vi "Auto_New.vi"() -> ()   [LabVIEW 2017]
uses:
  Control/Saurabh/prosucer_consumer_enum1.ctl
  Control/OUTPUT Cluster Indicator.ctl
  <vilib>/Utility/error.llb/DialogType.ctl
  <vilib>/addons/database/Connection.llb/DB Tools Open Connec (String).vi
  Global/DATA LOG.vi
  Global/Global 1.vi
  <vilib>/addons/database/NI_Database_API.lvlib
panel:
  out "SHIFT":string
  in  "BARCODE RECIPE":string(combo)
  out "PLC COM.":bool
  out "SHIFT_DATA":string[](array[string])
  out "stop":bool
  out "error out 2":errorcluster
  out "Shift 4":i32
  out "Time Stamp Out":timestamp[](array[timestamp]) format="%<%X>T"
  out "Time Stamp Out 4":timestamp[](array[timestamp]) format="%<%X>T"
  out "Shift_change":bool
  out "appended array":string[][](array[string])
  out "SHIFT_DATA 2":string[](array[string])
  in  "error in (no error)":errorcluster
  in  "Tab Control":enum32{"Screen 1", "Screen 2", "Daignostic"}(tab)
  out "OP 50":bool
  out "OP 40":bool
  out "OP 30":bool
  out "OP - 50":T1 {"RH Motor Screw" format="%#.2g N-m"; "LH Motor Screw" format="%#.2g N-m"; "Nut Torque" format="%#.2g N-m"}
  out "OP - 40":T2 {"Stack Load" format="%.2f kg"; "Dispalcement" format="%#.2g mm"; "LH Screw" format="%#.2g N-m"; "RH Screw" format="%#.2g N-m"}
  out "OP - 30":T3 {"Shaft Press Load" format="%#.2g kg"; "Displacement" format="%#.2g mm"}
  in  "stop 2":bool
  out "OP - 10":T4 {"Leak Rate" format="%#.2g SCCM"}
  in  "SIMULATE INPUT":bool[](array[boolean])=[FALSE, FALSE, FALSE, FALSE]
  out "OP - 20":T5 {"Top Load" format="%#.2g kg"; "Top Displace" format="%#.2g mm"; "Bottom Load" format="%#.2g kg"; "Bottom Displace" format="%#.2g mm"}
  out "OP 10 & 20":bool
  out "OP - 60":T6 {"Screw 6" format="%#.2g N-m"; "Screw 5" format="%#.2g N-m"; "Screw 4" format="%#.2g N-m"; "Screw 3" format="%#.2g N-m"; "Screw 2" format="%#.2g N-m"; "Screw 1" format="%#.2g N-m"}
  out "OP - 70":T7 {"Full Open" format="%#.4g V"; "Full Close" format="%#.4g V"}
  out "OP - 110":cluster{"BARCODE":string}
  out "OP - 80":T8 {"Plug Press Load" format="%#.2f kg"}
  out "OP - 90":T9 {"Steam Leak" format="%#_g sccm"; "Seat Leak" format="%#_g LPM"}
  out "OP - 100":T10 {"Response Time REV" format="%#_g msec"; "Response time FWD" format="%#_g msec"; "Motor Full Open" format="%#.2f V"; "Motor Start Back" format="%#.2f V"; "Motor Full Close" format="%#.2f V"; "Motor Start Of Close" format="%#.2f V"; "Motor Peak" format="%#.2f A"; "Sensor O/P Full Close" format="%#.2f V"; "Sensor O/P Start Of Close" format="%#.2f V"; "Sensor O/P Open" format="%#.2f V"}
  out "OP 60":bool
  out "OP 70 & 80":bool
  out "OP 90 -100 - 110":bool
  out "OP110 STATUS":dbl[](array[numeric])
  out "SCAN OP110":string[](array[string])
  out "OP100 STATUS":dbl[](array[numeric])
  out "SCAN OP100":string[](array[string])
  out "OP50 STATUS":dbl[](array[numeric])
  out "SCAN OP50":string[](array[string])
  out "OP90 STATUS":dbl[](array[numeric])
  out "SCAN OP90":string[](array[string])
  out "OP80 STATUS":dbl[](array[numeric])
  out "SCAN OP80":string[](array[string])
  out "OP70 STATUS":dbl[](array[numeric])
  out "SCAN OP70":string[](array[string])
  out "OP60 STATUS":dbl[](array[numeric])
  out "SCAN OP60":string[](array[string])
  out "OP40 STATUS":dbl[](array[numeric])
  out "SCAN OP40":string[](array[string])
  out "OP30 STATUS":dbl[](array[numeric])
  out "SCAN OP30":string[](array[string])
  out "OP20 STATUS":dbl[](array[numeric])
  out "SCAN OP20":string[](array[string])
  out "OP10 STATUS":dbl[](array[numeric])
  out "SCAN OP10":string[](array[string])
  # "Op10 20\nOp30\nOp 40\nOp50\nOp60\nOp70-80\nOp 90-100-110"
  # "SENSOR MIN VLTG"
  # "OP - 50"
  # "OP - 40"
  # "OP - 30"
  # "OP - 10"
  # "OP - 20"
  # "OP - 60"
  # "OP - 70"
  # "OP - 110"
  # "OP - 80"
  # "OP - 90"
  # "OP - 100"
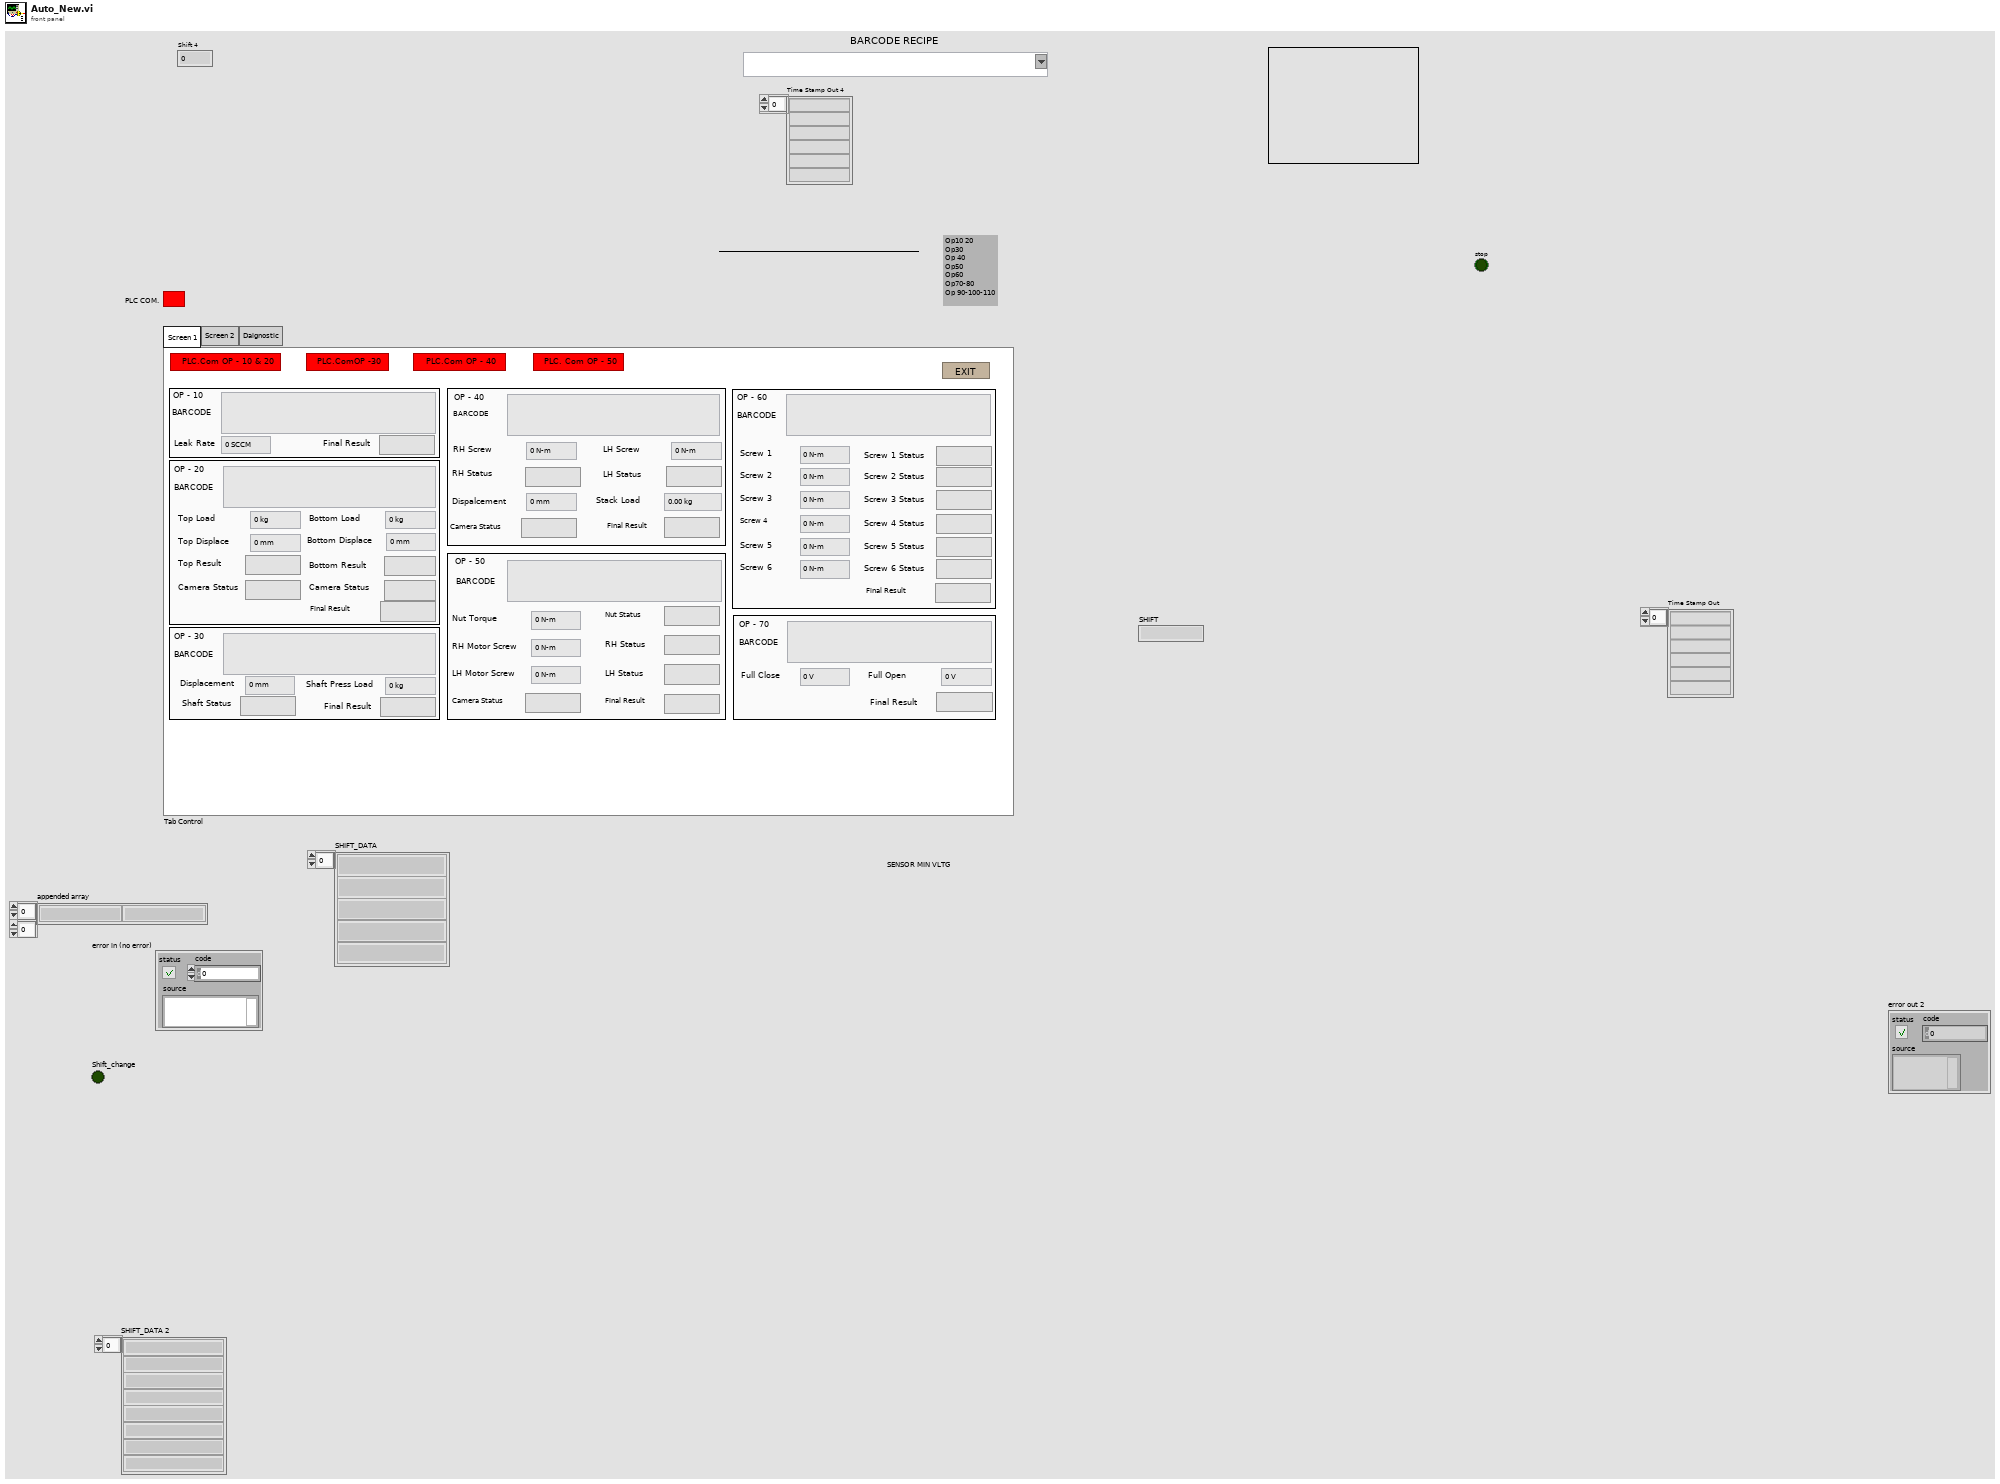
[diagram p1: front panel]
types:
  T1 = cluster{"BARCODE":string, "Nut Torque":dbl, "LH Motor Screw":dbl, "LH Status":bool, "RH Status":bool, "RH Motor Screw":dbl, "Final Result":bool, "Nut Status":bool, "Camera Status":bool}
  T2 = cluster{"BARCODE":string, "RH Screw":dbl, "LH Screw ":dbl, "RH Status":bool, "LH Status":bool, "Dispalcement ":dbl, "Stack Load ":dbl, "Final Result":bool, "Camera Status":bool}
  T3 = cluster{"BARCODE":string, "Displacement":dbl, "Shaft Press Load":dbl, "Shaft Status":bool, "Final Result":bool}
  T4 = cluster{"BARCODE":string, "Leak Rate":dbl, "Final Result":bool}
  T5 = cluster{"BARCODE":string, "Bottom Displace":dbl, "Bottom Load":dbl, "Camera Status":bool, "Bottom Result":bool, "Top Displace":dbl, "Top Load ":dbl, "Camera Status":bool, "Top Result":bool, "Final Result":bool}
  T6 = cluster{"BARCODE":string, "Screw 1":dbl, "Screw 2":dbl, "Screw 1 Status":bool, "Screw 2 Status":bool, "Screw 3":dbl, "Final Result":bool, "Screw 3 Status":bool, "Screw 4":dbl, "Screw 5":dbl, "Screw 4 Status":bool, "Screw 5 Status":bool, "Screw 6":dbl, "Screw 6 Status":bool}
  T7 = cluster{"BARCODE":string, "Full Close":dbl, "Full Open":dbl, "Final Result":bool}
  T8 = cluster{"BARCODE":string, "Plug Press Load":dbl, "Final Result":bool, "Loctite Status":bool}
  T9 = cluster{"BARCODE":string, "Seat Leak":dbl, "Seat Status":bool, "Steam Leak":dbl, "Final Result":bool}
  T10 = cluster{"BARCODE":string, "Sensor O/P Open":dbl, "Sensor O/P Start Of Close":dbl, "Final Result":bool, "Sensor O/P Full Close":dbl, "Motor Peak":dbl, "Motor Start Of Close":dbl, "Motor Full Close":dbl, "Motor Start Back":dbl, "Motor Full Open":dbl, "Response time FWD":dbl, "Response Time REV":dbl, "Camera Status":bool}
  T11 = typedef "OUTPUT Cluster Indicator.ctl" = cluster{"OP - 10":cluster{"BARCODE":string, "LEAK RATE":dbl, "RESULT":bool}, "OP - 30":cluster{"BARCODE":string, "Displacement":dbl, "Load":dbl, "Middle Gear Shaft Status":bool, "Final Result":bool}, "OP - 60":cluster{"BARCODE":string, "Screw 1 Data":dbl, "Screw 2 data":dbl, "Screw 1 Status":bool, "Screw 2 Status":bool, "Screw3 Data":dbl, "Final Result":bool, "Screw3 Status":bool, "Screw4 Data":dbl, "Screw5 Data":dbl, "Screw4 Status":bool, "Screw5 Status":bool, "Screw6 Data":dbl, "Screw6 Status":bool}, "OP - 70":cluster{"BARCODE":string, "Sensor MIN Vltg":dbl, "Sensor MAX Vltg":dbl, "Final Result":bool}, "OP - 80":cluster{"BARCODE":string, "Load":dbl, "Final Result":bool, "Dispensing":bool}, "OP - 90":cluster{"BARCODE":string, "Seat LT Data":dbl, "Seat Status":bool, "Steam LT Data":dbl, "Final Result":bool}, "OP - 110":cluster{"BARCODE":string}, "OP - 20":cluster{"BARCODE":string, "Bottom Displace":dbl, "Bottom Load":dbl, "Camera Status":bool, "Bottom Result":bool, "Top Displace":dbl, "Top Load ":dbl, "Camera Status":bool, "Top Result":bool, "Final Result":bool}, "OP - 50":cluster{"BARCODE":string, "Nut Torque":dbl, "LH Motor Screw":dbl, "LH Status":bool, "RH Status":bool, "RH Motor Screw":dbl, "Final Result":bool, "Nut Status":bool, "Camera Status":bool}, "OP - 100":cluster{"BARCODE":string, "Sensor O/P Open":dbl, "Sensor O/P Start Of Close":dbl, "Final Result":bool, "Sensor O/P Full Close":dbl, "Motor Peak":dbl, "Motor Start Of Close":dbl, "Motor Full Close":dbl, "Motor Start Back":dbl, "Motor Full Open":dbl, "Response time FWD":dbl, "Response Time REV":dbl, "Camera Status":bool}, "OP - 40":cluster{"BARCODE":string, "RH Screw":dbl, "LH Screw ":dbl, "RH Status":bool, "LH Status":bool, "Dispalcement ":dbl, "Stack Load ":dbl, "Final Result":bool, "Camera Status":bool}}
  T12 = cluster{"OP - 10":cluster{"BARCODE":string, "LEAK RATE":dbl, "RESULT":bool}, "OP - 30":cluster{"BARCODE":string, "Displacement":dbl, "Load":dbl, "Middle Gear Shaft Status":bool, "Final Result":bool}, "OP - 60":cluster{"BARCODE":string, "Screw 1 Data":dbl, "Screw 2 data":dbl, "Screw 1 Status":bool, "Screw 2 Status":bool, "Screw3 Data":dbl, "Final Result":bool, "Screw3 Status":bool, "Screw4 Data":dbl, "Screw5 Data":dbl, "Screw4 Status":bool, "Screw5 Status":bool, "Screw6 Data":dbl, "Screw6 Status":bool}, "OP - 70":cluster{"BARCODE":string, "Sensor MIN Vltg":dbl, "Sensor MAX Vltg":dbl, "Final Result":bool}, "OP - 80":cluster{"BARCODE":string, "Load":dbl, "Final Result":bool, "Dispensing":bool}, "OP - 90":cluster{"BARCODE":string, "Seat LT Data":dbl, "Seat Status":bool, "Steam LT Data":dbl, "Final Result":bool}, "OP - 110":cluster{"BARCODE":string}, "OP - 20":cluster{"BARCODE":string, "Bottom Displace":dbl, "Bottom Load":dbl, "Camera Status":bool, "Bottom Result":bool, "Top Displace":dbl, "Top Load ":dbl, "Camera Status":bool, "Top Result":bool, "Final Result":bool}, "OP - 40":cluster{"BARCODE":string, "RH Screw":dbl, "LH Screw ":dbl, "RH Status":bool, "LH Status":bool, "Dispalcement ":dbl, "Stack Load ":dbl, "Final Result":bool}, "OP - 50":cluster{"BARCODE":string, "Nut Torque":dbl, "LH Motor Screw":dbl, "LH Status":bool, "RH Status":bool, "RH Motor Screw":dbl, "Final Result":bool, "Nut Status":bool, "Camera Status":bool}, "OP - 100":cluster{"BARCODE":string, "Sensor O/P Open":dbl, "Sensor O/P Start Of Close":dbl, "Final Result":bool, "Sensor O/P Full Close":dbl, "Motor Peak":dbl, "Motor Start Of Close":dbl, "Motor Full Close":dbl, "Motor Start Back":dbl, "Motor Full Open":dbl, "Response time FWD":dbl, "Response Time REV":dbl, "Camera Status":bool}}
  T13 = typedef "prosucer_consumer_enum1.ctl" = enum16{"-1", "SCAN1", "SCAN2", "SCAN3", "SCAN4", "SCAN5", "SCAN6", "SCAN7", "SCAN8", "SCAN9", "SCAN10", "SCAN11", "STOP", "DATALOG1", "DATALOG2", "DATALOG3", "DATALOG4", "DATALOG5", "DATALOG6", "DATALOG7", "DATALOG8", "DATALOG9", "DATALOG10", "DATALOG11", "CYCLE_START1", "CYCLE_START2", "CYCLE_START3", "CYCLE_START4", "BARCODE RECIPE", "EMERGENCY STOP"}
  T14 = typedef "NI_Database_API.lvlib/Conn ObjectReference.ctl" = refnum<k1>
  T15 = typedef "DialogType.ctl" = u16
  T16 = cluster{"trimmed string":string, "SHIFT":string, "date/time string":string, string, "Input 2":string}
  T17 = cluster{"SHIFT":string, "date/time string":string, "Input 2":string, string}
  T18 = cluster{"date/time string":string, "Input 2":string, "Input 2":string, "Input 2":string, "Input 2":string, "Input 2":string, "Input 2":string, "Input 2":string, "Input 2":string, "Input 2":string, "Input 2":string}
  T19 = cluster{"date/time string":string, "SHIFT":string, "Input 2":string, "Input 2":string, "Input 2":string, "Input 2":string, "Input 2":string, "Input 2":string, "Input 2":string, "Input 2":string, "Input 2":string, "Input 2":string}
  T20 = cluster{"date/time string":string, "Input 2":string, "Input 2":string, "Input 2":string, "Input 2":string}
  T21 = cluster{"date/time string":string, "SHIFT":string, "Input 2":string, "Input 2":string, "Input 2":string, "Input 2":string}
  T22 = cluster{"date/time string":string, "Input 2":string, "Input 2":string, "Input 2":string, "Input 2":string, "Input 2":string, "Input 2":string, "Input 2":string, "Input 2":string}
  T23 = cluster{"date/time string":string, "SHIFT":string, "Input 2":string, "Input 2":string, "Input 2":string, "Input 2":string, "Input 2":string, "Input 2":string, "Input 2":string, "Input 2":string}
  T24 = cluster{"date/time string":string, "SHIFT":string, "Input 2":string, "Input 2":string, "Input 2":string, "Input 2":string, "Input 2":string, "Input 2":string}
  T25 = cluster{"date/time string":string, "Input 2":string, "Input 2":string, "Input 2":string, "Input 2":string, "Input 2":string, "Input 2":string, "Input 2":string, "Input 2":string, "Input 2":string, "Input 2":string, "Input 2":string, "Input 2":string, "Input 2":string}
  T26 = cluster{"date/time string":string, "SHIFT":string, "Input 2":string, "Input 2":string, "Input 2":string, "Input 2":string, "Input 2":string, "Input 2":string, "Input 2":string, "Input 2":string, "Input 2":string, "Input 2":string, "Input 2":string, "Input 2":string}
  T27 = cluster{"date/time string":string, "Input 2":string, "Input 2":string, "Input 2":string}
  T28 = cluster{"date/time string":string, "SHIFT":string, "Input 2":string, "Input 2":string, "Input 2":string}
  T29 = cluster{"Input 2":string, "SHIFT":string, "date/time string":string, "Input 2":string, "Input 2":string, "Input 2":string}
  T30 = cluster{"BARCODE":string, "Seat LT Data":dbl, "Seat Status":bool, "Steam LT Data":dbl, "Final Result":bool}
  T31 = cluster{"BARCODE":string, "LEAK RATE":dbl, "RESULT":bool}
  T32 = cluster{"BARCODE":string, "Displacement":dbl, "Load":dbl, "Middle Gear Shaft Status":bool, "Final Result":bool}
  T33 = cluster{"BARCODE":string, "Screw 1 Data":dbl, "Screw 2 data":dbl, "Screw 1 Status":bool, "Screw 2 Status":bool, "Screw3 Data":dbl, "Final Result":bool, "Screw3 Status":bool, "Screw4 Data":dbl, "Screw5 Data":dbl, "Screw4 Status":bool, "Screw5 Status":bool, "Screw6 Data":dbl, "Screw6 Status":bool}
  T34 = cluster{"BARCODE":string, "Sensor MIN Vltg":dbl, "Sensor MAX Vltg":dbl, "Final Result":bool}
  T35 = cluster{"BARCODE":string, "Load":dbl, "Final Result":bool, "Dispensing":bool}
  T36 = enum32{"invalid app kind", "Development System", "Run Time System", "Student Edition", "Embedded LabVIEW", "Evaluation", "Custom"}
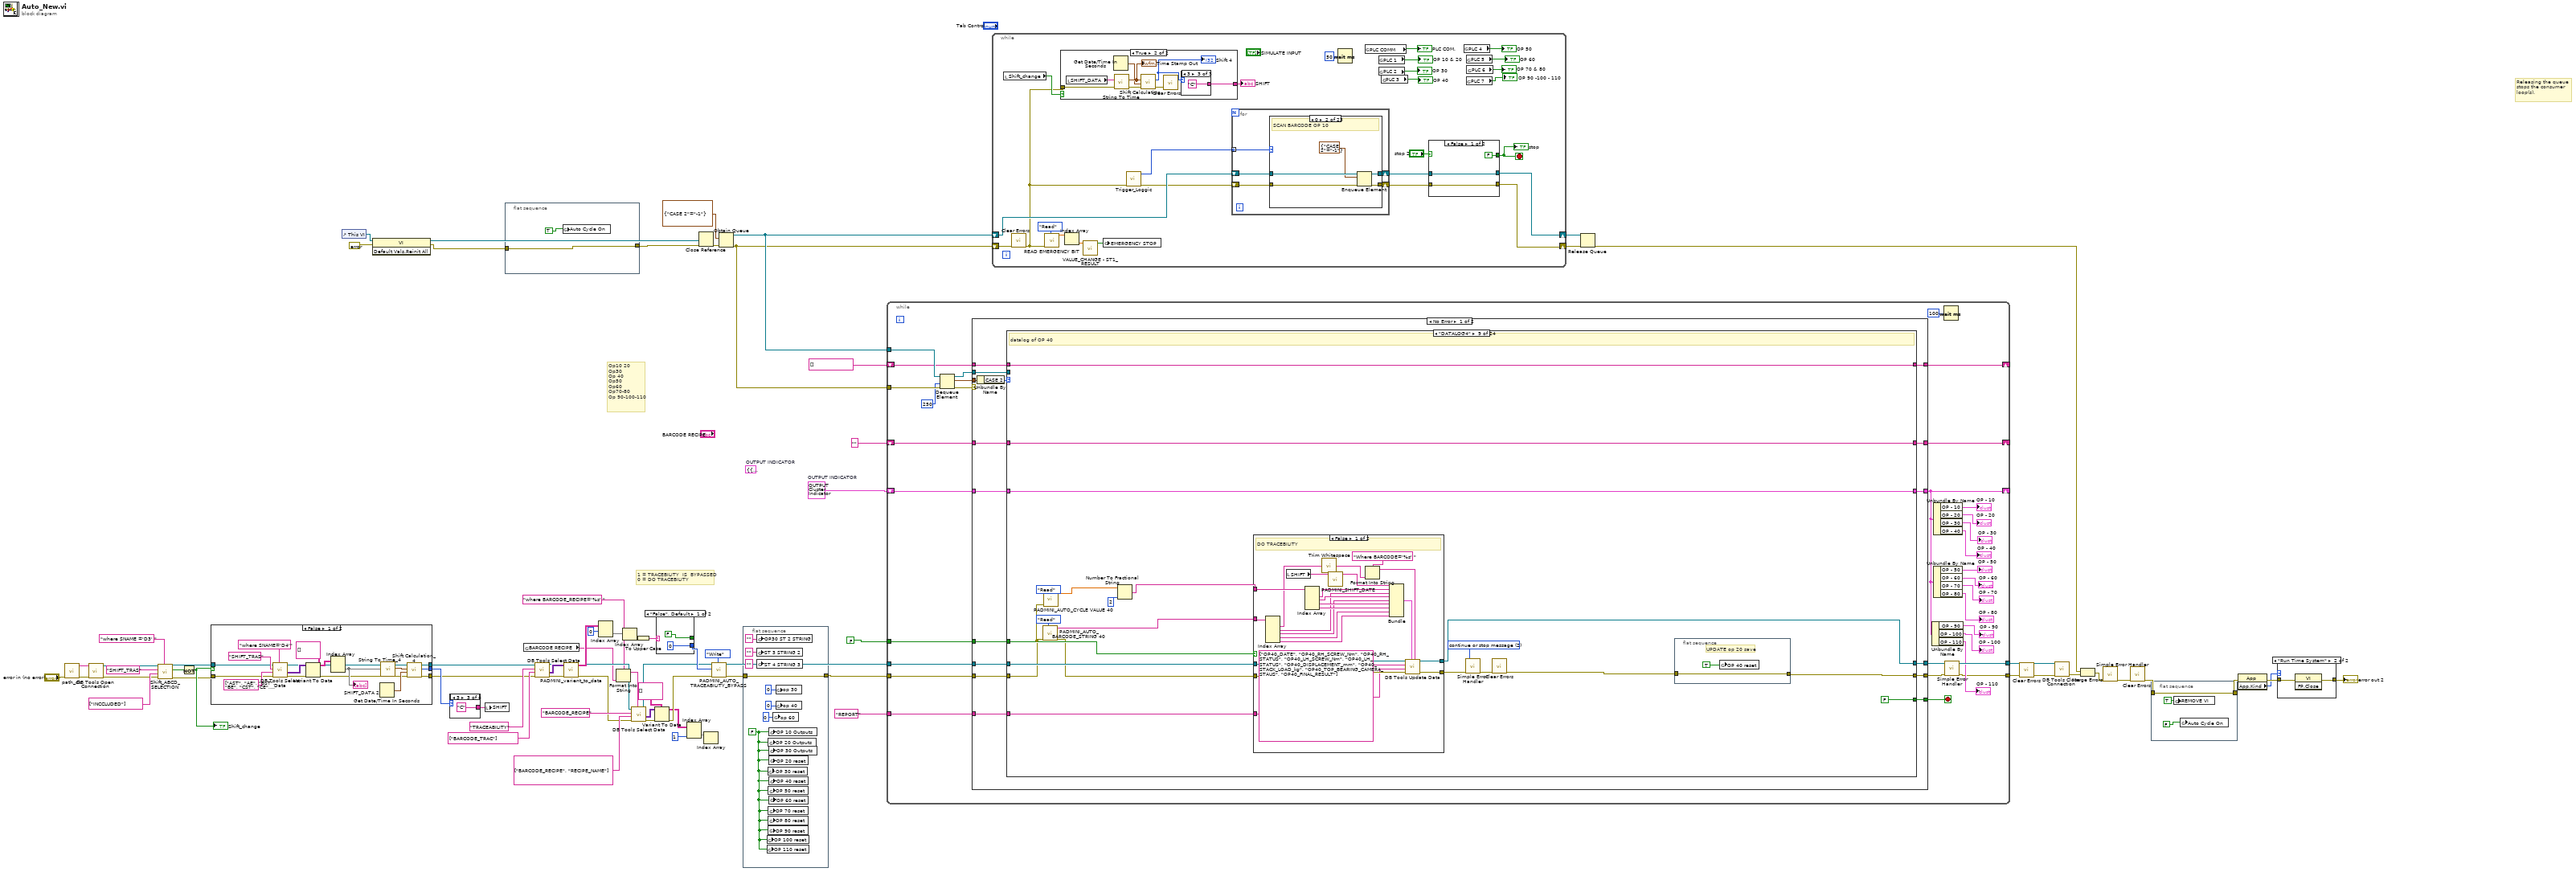
[diagram p0: block diagram]
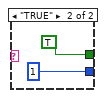
[diagram p2: hidden frame]
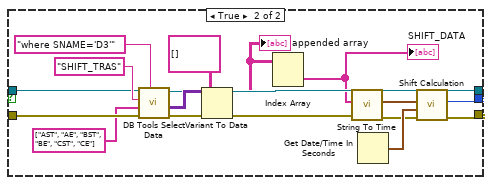
[diagram p3: hidden frame]
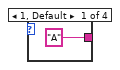
[diagram p4: hidden frame]
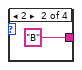
[diagram p5: hidden frame]
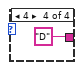
[diagram p6: hidden frame]
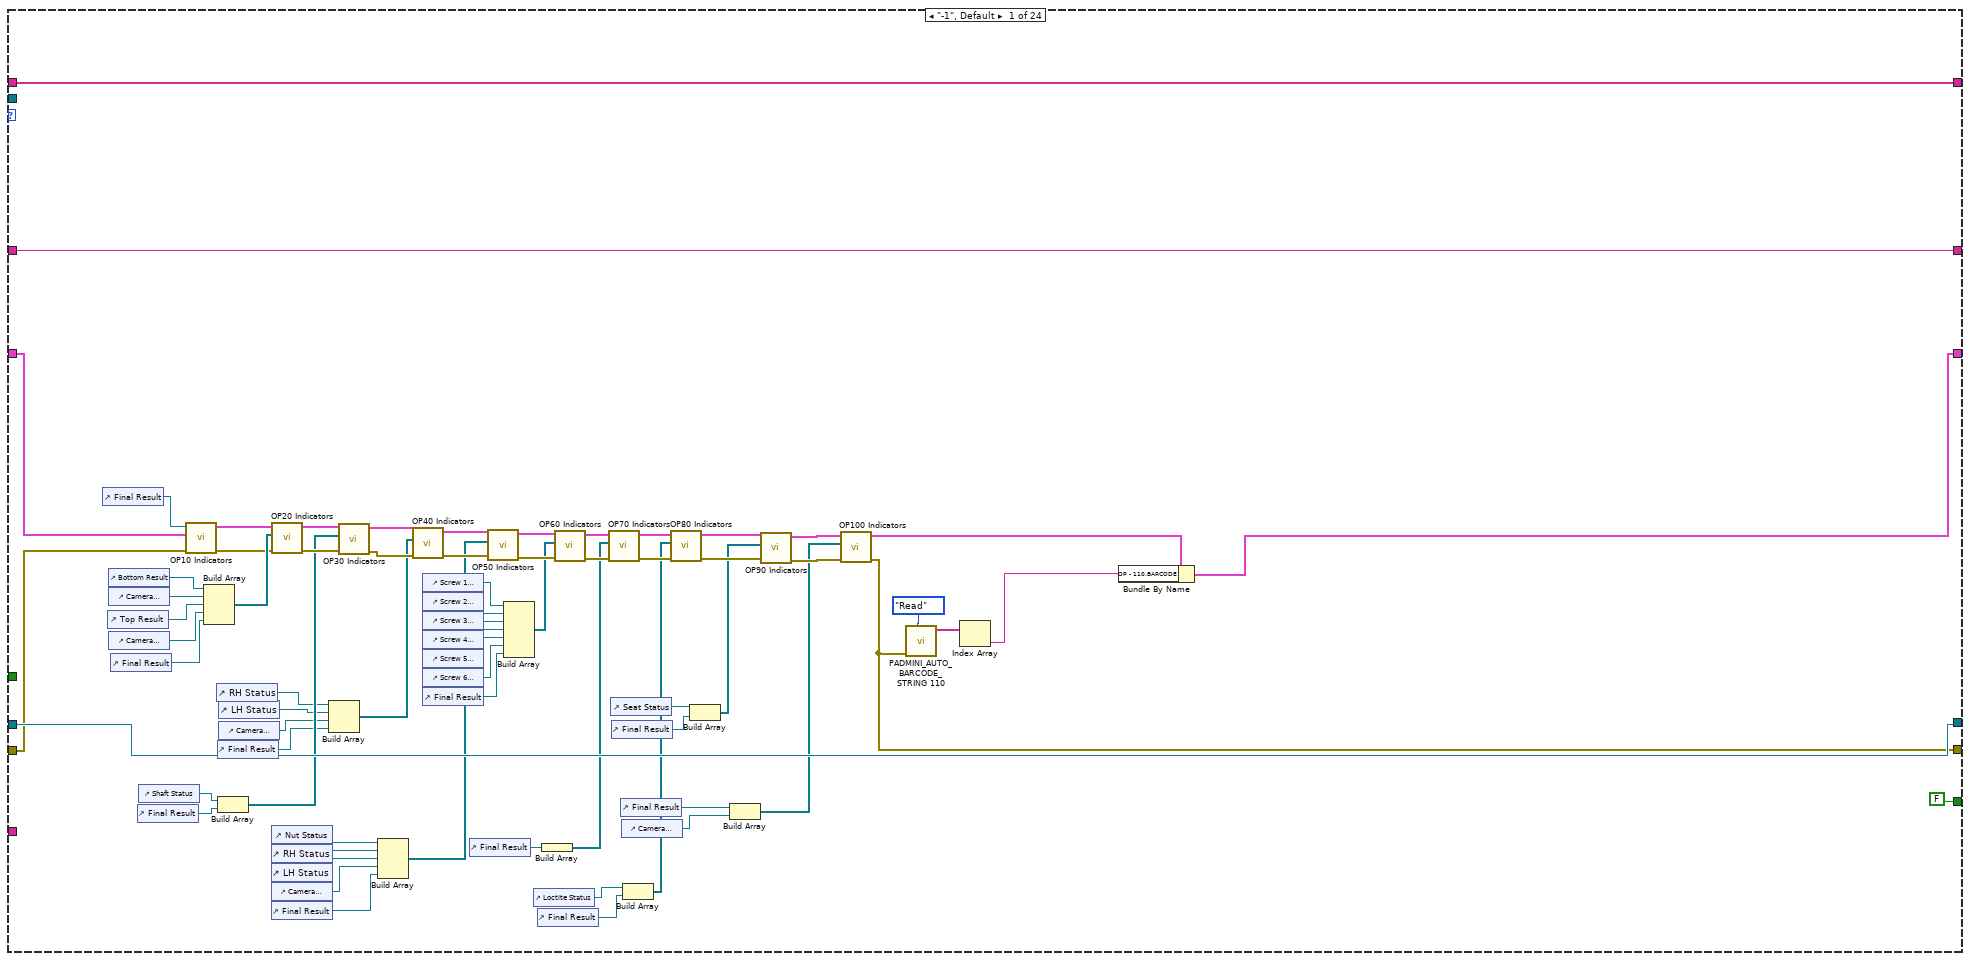
[diagram p7: hidden frame]
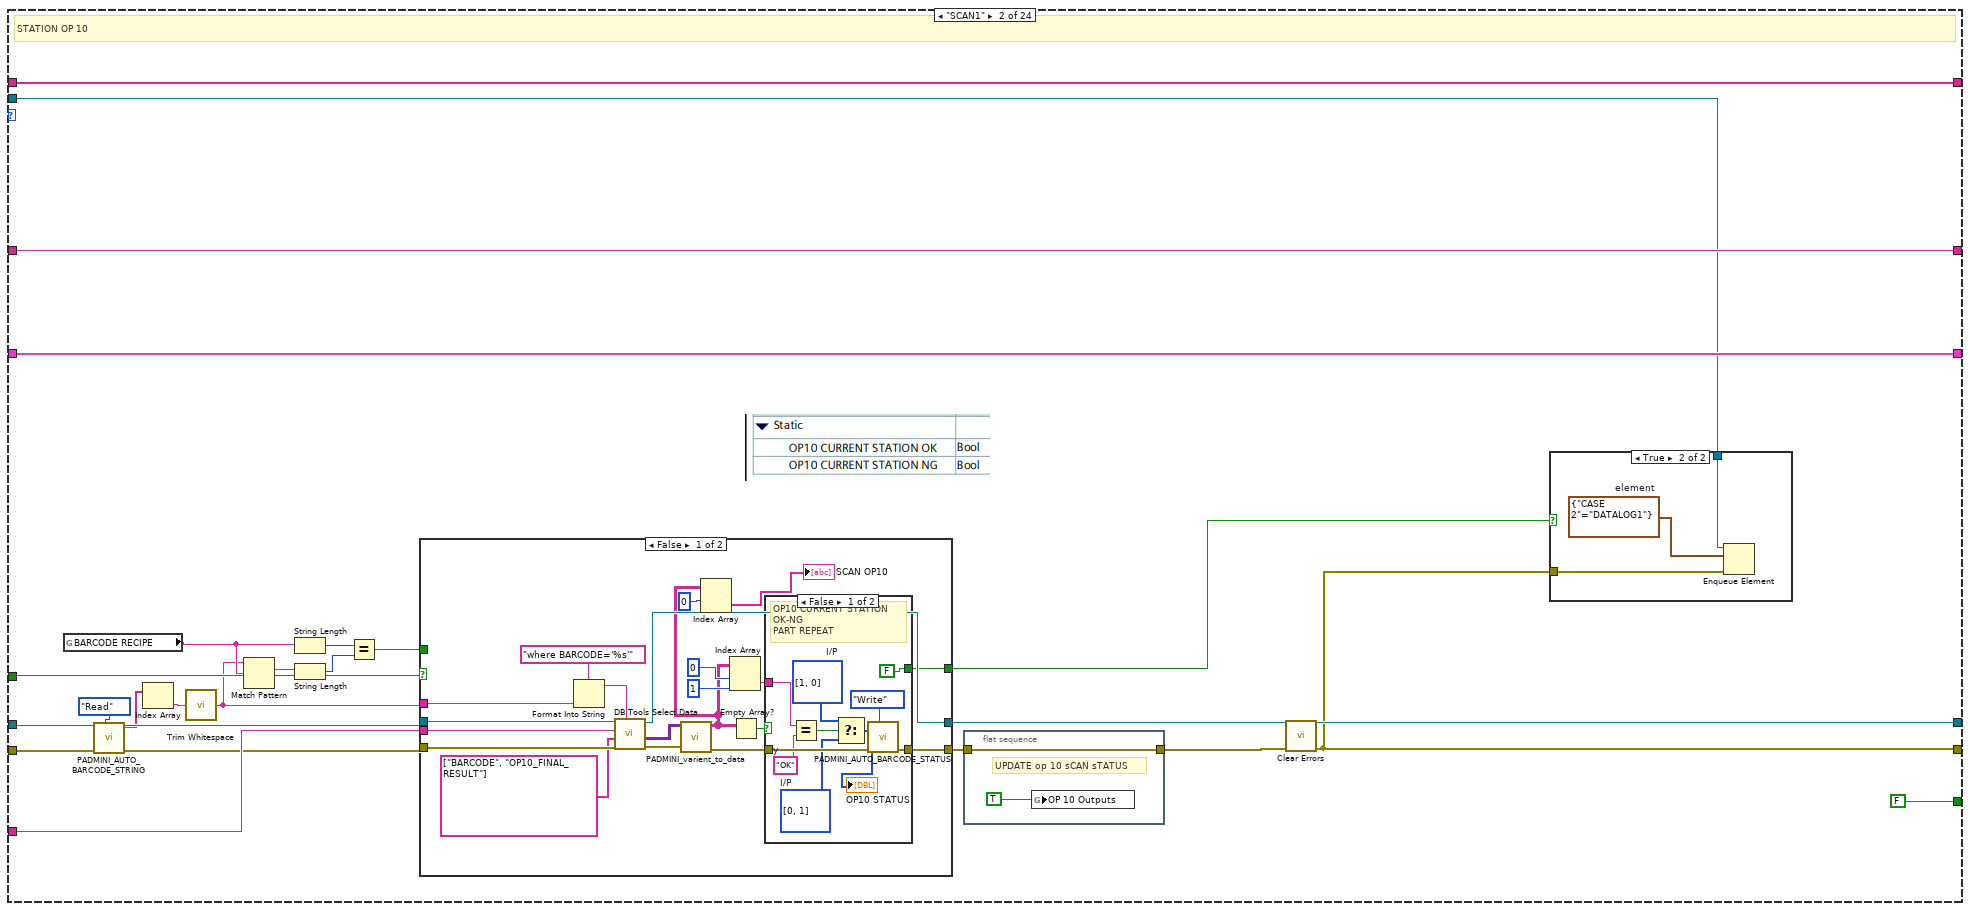
[diagram p8: hidden frame]
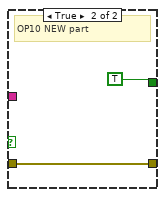
[diagram p10: hidden frame]
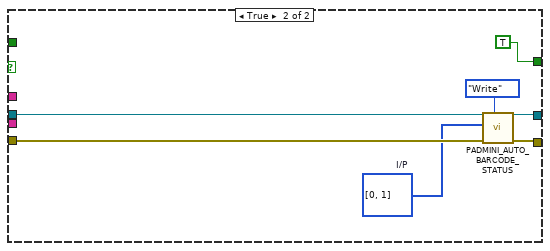
[diagram p11: hidden frame]
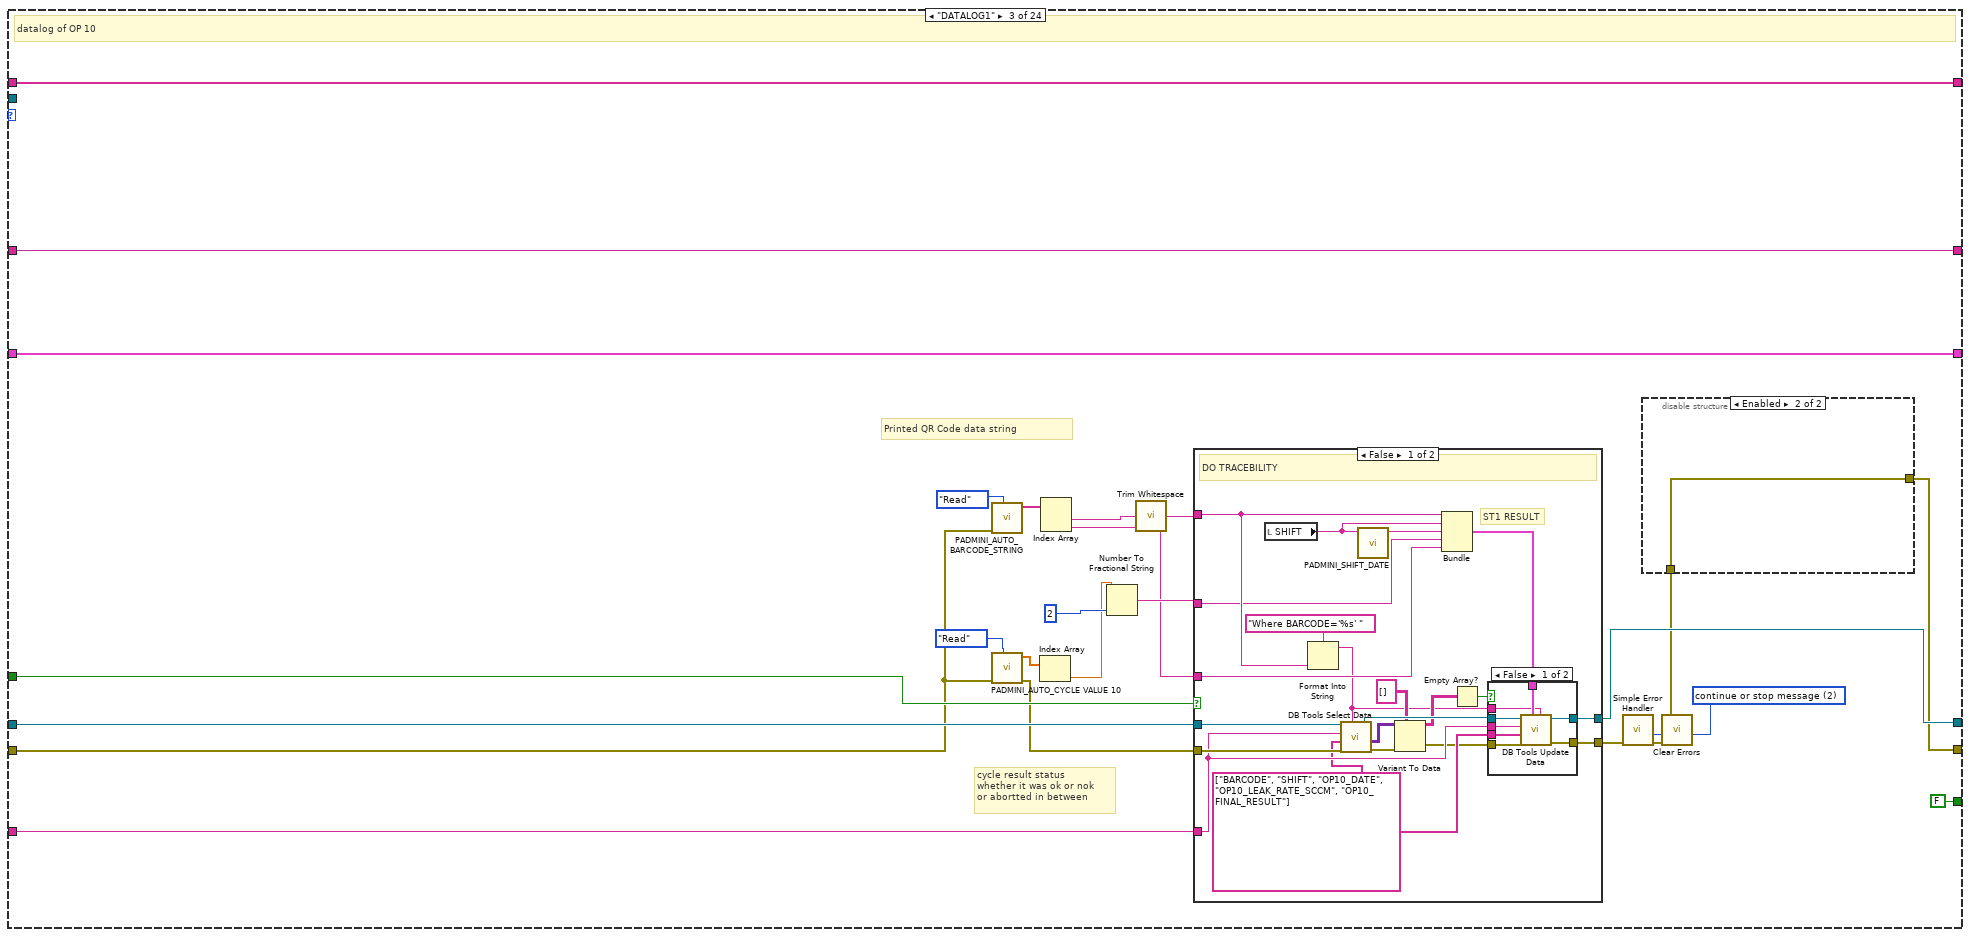
[diagram p12: hidden frame]
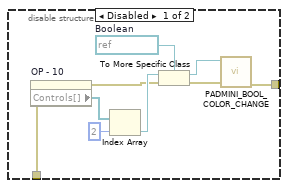
[diagram p13: hidden frame]
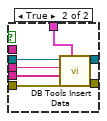
[diagram p14: hidden frame]
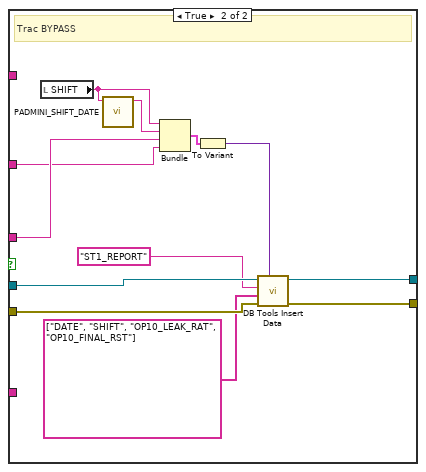
[diagram p15: hidden frame]
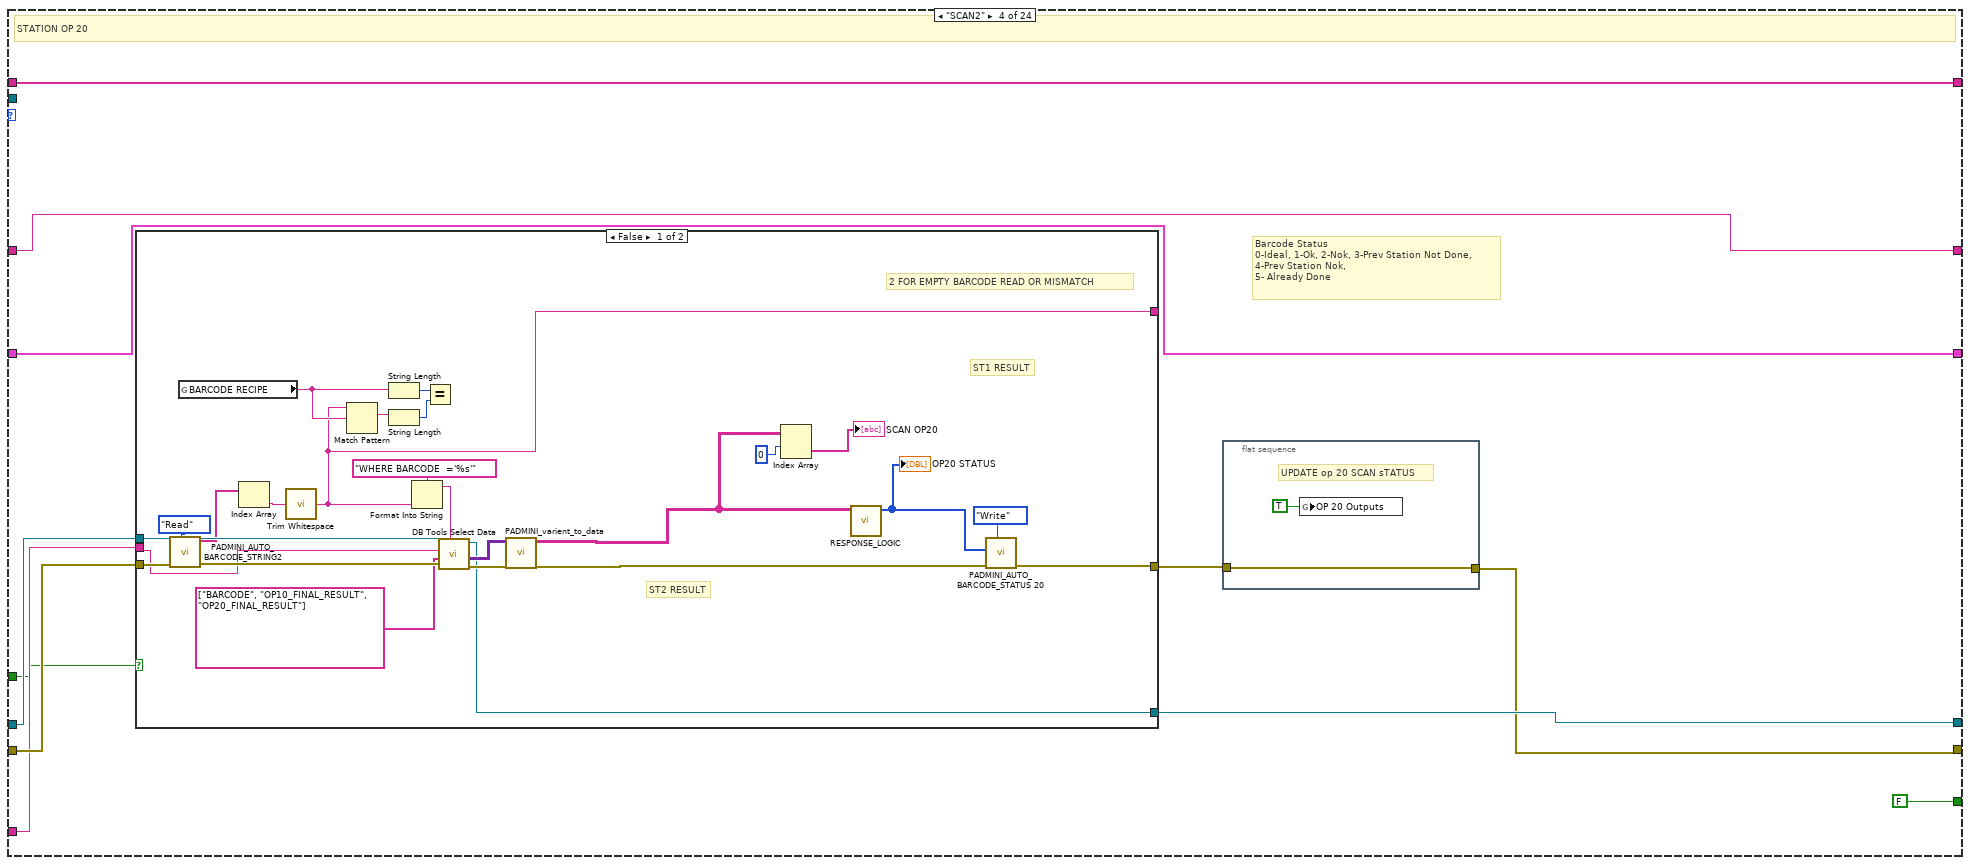
[diagram p16: hidden frame]
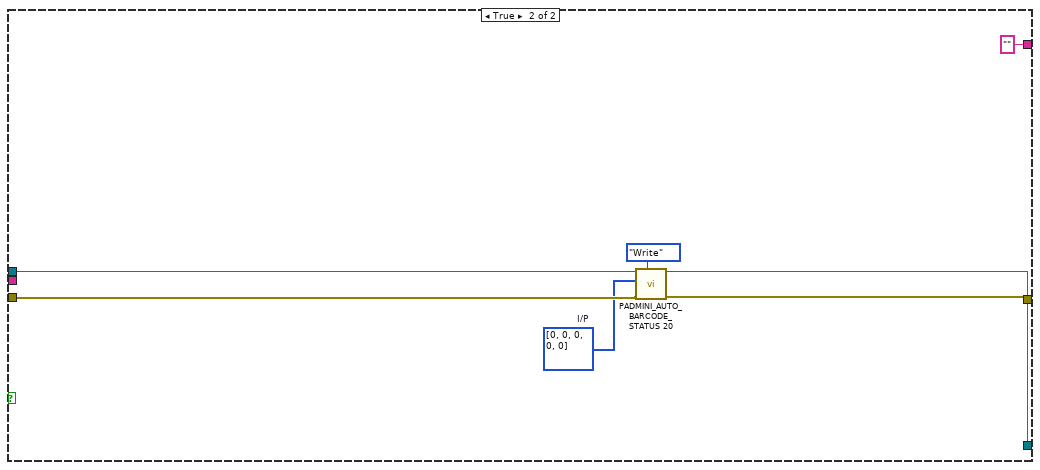
[diagram p17: hidden frame]
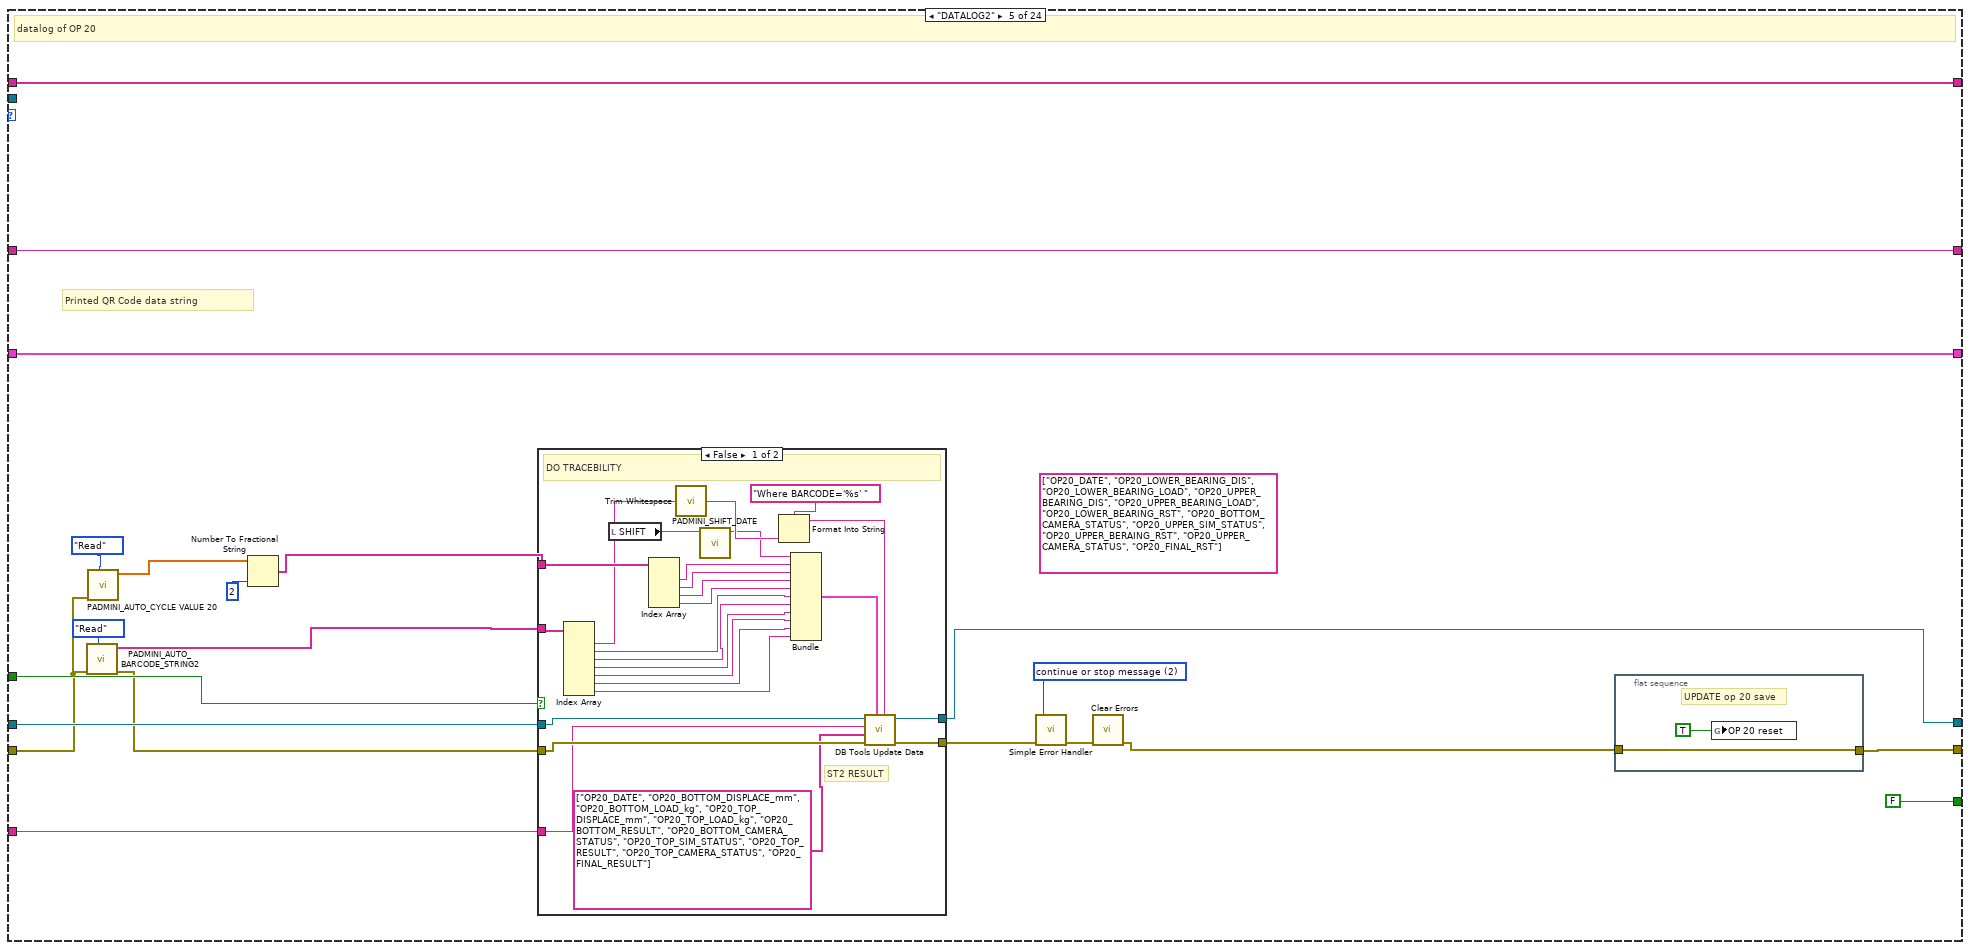
[diagram p18: hidden frame]
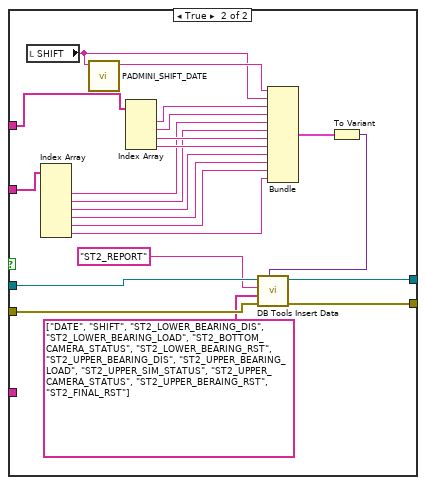
[diagram p19: hidden frame]
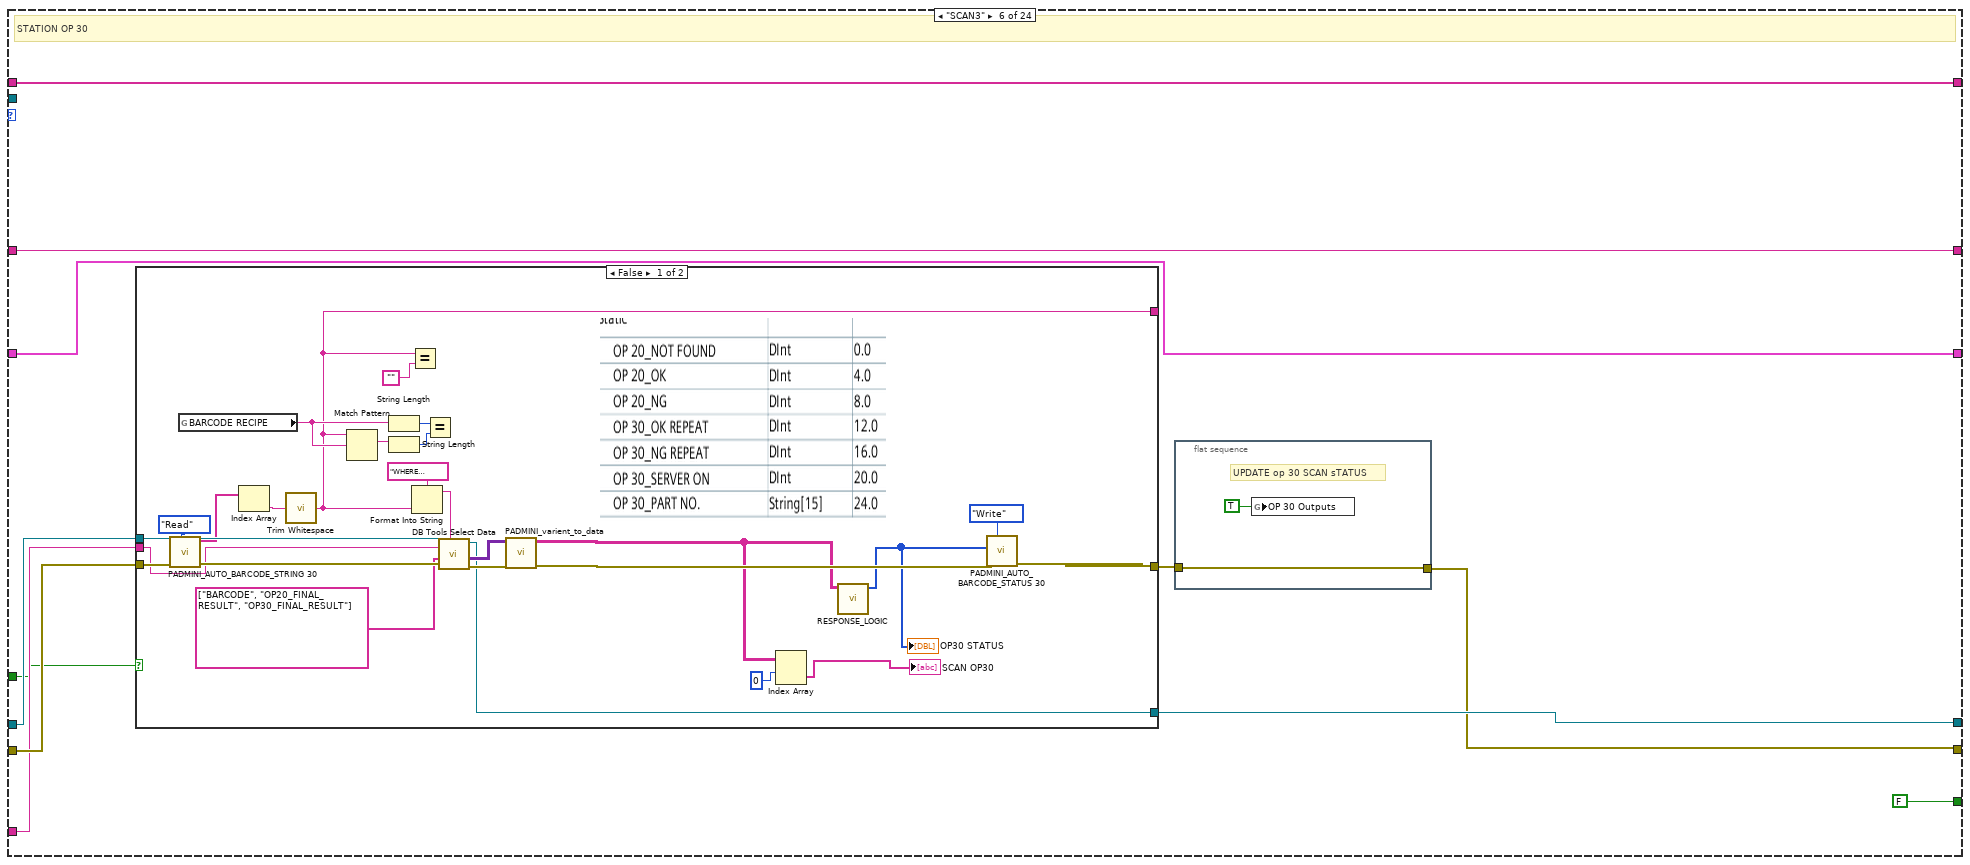
[diagram p20: hidden frame]
diagram:
  w1 = T11 {"OP - 10"={"BARCODE"="", "LEAK RATE"=0.0, "RESULT"=FALSE}, "OP - 30"={"BARCODE"="", "Displacement"=0.0, "Load"=0.0, "Middle Gear Shaft Status"=FALSE, "Final Result"=FALSE}, "OP - 60"={"BARCODE"="", "Screw 1 Data"=0.0, "Screw 2 data"=0.0, "Screw 1 Status"=FALSE, "Screw 2 Status"=FALSE, "Screw3 Data"=0.0, "Final Result"=FALSE, "Screw3 Status"=FALSE, "Screw4 Data"=0.0, "Screw5 Data"=0.0, "Screw4 Status"=FALSE, "Screw5 Status"=FALSE, "Screw6 Data"=0.0, "Screw6 Status"=FALSE}, "OP - 70"={"BARCODE"="", "Sensor MIN Vltg"=0.0, "Sensor MAX Vltg"=0.0, "Final Result"=FALSE}, "OP - 80"={"BARCODE"="", "Load"=0.0, "Final Result"=FALSE, "Dispensing"=FALSE}, "OP - 90"={"BARCODE"="", "Seat LT Data"=0.0, "Seat Status"=FALSE, "Steam LT Data"=0.0, "Final Result"=FALSE}, "OP - 110"={"BARCODE"=""}, "OP - 20"={"BARCODE"="", "Bottom Displace"=0.0, "Bottom Load"=0.0, "Camera Status"=FALSE, "Bottom Result"=TRUE, "Top Displace"=0.0, "Top Load "=0.0, "Camera Status"=FALSE, "Top Result"=FALSE, "Final Result"=FALSE}, "OP - 50"={"BARCODE"="", "Nut Torque"=0.0, "LH Motor Screw"=0.0, "LH Status"=FALSE, "RH Status"=FALSE, "RH Motor Screw"=0.0, "Final Result"=FALSE, "Nut Status"=FALSE, "Camera Status"=FALSE}, "OP - 100"={"BARCODE"="", "Sensor O/P Open"=0.0, "Sensor O/P Start Of Close"=0.0, "Final Result"=FALSE, "Sensor O/P Full Close"=0.0, "Motor Peak"=0.0, "Motor Start Of Close"=0.0, "Motor Full Close"=0.0, "Motor Start Back"=0.0, "Motor Full Open"=0.0, "Response time FWD"=0.0, "Response Time REV"=0.0, "Camera Status"=FALSE}, "OP - 40"={"BARCODE"="", "RH Screw"=0.0, "LH Screw "=0.0, "RH Status"=FALSE, "LH Status"=FALSE, "Dispalcement "=0.0, "Stack Load "=0.0, "Final Result"=FALSE, "Camera Status"=TRUE}}  # OUTPUT INDICATOR
  (unwired) T12 {"OP - 10"={"BARCODE"="", "LEAK RATE"=0.0, "RESULT"=FALSE}, "OP - 30"={"BARCODE"="", "Displacement"=0.0, "Load"=0.0, "Middle Gear Shaft Status"=FALSE, "Final Result"=FALSE}, "OP - 60"={"BARCODE"="", "Screw 1 Data"=0.0, "Screw 2 data"=0.0, "Screw 1 Status"=FALSE, "Screw 2 Status"=FALSE, "Screw3 Data"=0.0, "Final Result"=FALSE, "Screw3 Status"=FALSE, "Screw4 Data"=0.0, "Screw5 Data"=0.0, "Screw4 Status"=FALSE, "Screw5 Status"=FALSE, "Screw6 Data"=0.0, "Screw6 Status"=FALSE}, "OP - 70"={"BARCODE"="", "Sensor MIN Vltg"=0.0, "Sensor MAX Vltg"=0.0, "Final Result"=FALSE}, "OP - 80"={"BARCODE"="", "Load"=0.0, "Final Result"=FALSE, "Dispensing"=FALSE}, "OP - 90"={"BARCODE"="", "Seat LT Data"=0.0, "Seat Status"=FALSE, "Steam LT Data"=0.0, "Final Result"=FALSE}, "OP - 110"={"BARCODE"=""}, "OP - 20"={"BARCODE"="", "Bottom Displace"=0.0, "Bottom Load"=0.0, "Camera Status"=FALSE, "Bottom Result"=TRUE, "Top Displace"=0.0, "Top Load "=0.0, "Camera Status"=FALSE, "Top Result"=FALSE, "Final Result"=FALSE}, "OP - 40"={"BARCODE"="", "RH Screw"=0.0, "LH Screw "=0.0, "RH Status"=FALSE, "LH Status"=FALSE, "Dispalcement "=0.0, "Stack Load "=0.0, "Final Result"=FALSE}, "OP - 50"={"BARCODE"="", "Nut Torque"=0.0, "LH Motor Screw"=0.0, "LH Status"=FALSE, "RH Status"=FALSE, "RH Motor Screw"=0.0, "Final Result"=FALSE, "Nut Status"=FALSE, "Camera Status"=FALSE}, "OP - 100"={"BARCODE"="", "Sensor O/P Open"=0.0, "Sensor O/P Start Of Close"=0.0, "Final Result"=FALSE, "Sensor O/P Full Close"=0.0, "Motor Peak"=0.0, "Motor Start Of Close"=0.0, "Motor Full Close"=0.0, "Motor Start Back"=0.0, "Motor Full Open"=0.0, "Response time FWD"=0.0, "Response Time REV"=0.0, "Camera Status"=FALSE}}  # OUTPUT INDICATOR
  # "Op10 20\nOp30\nOp 40\nOp50\nOp60\nOp70-80\nOp 90-100-110"
  # "1 = TRACEBILITY  IS  BYPASSED\n0 = DO TRACEBILITY"
  # "Releasing the queue stops the consumer loop(s)."
  n1 = call "path_db.vi"("error in"="error in (no error)") -> ("error out"=w48:errorcluster, "resulting string"=w69:string)  [unwired: 9 in]
  n2 = call-poly <vilib>:"DB Tools Open Connection.vi"("error in (no error)"=w48, "connection information"=w69) -> ("error out"=w47:errorcluster, "connection reference"=w41:T14)  [unwired: 6 in]
  n3 = call "Shift_ABCD_SELECTION.vi"("Where"="where SNAME ='D3' ", "error in (no error)"=w47, "Array"=string[] ["INCCLUDED"], "table"="SHIFT_TRAS", "Refnum in"=w41) -> ("error out"=w5:errorcluster, "Boolean"=w60:bool, "Refnum out"=w61:T14)  [unwired: 4 in]
  n4 = Not(x=w60) -> (.not. x?=w59:bool)
  "Shift_change" <- w59
  n5 = case shown="False" w59 {
    tunnel: [w74 w98] -> w65
    tunnel: w61 -> [w77 w96]
    tunnel: w5 -> [w76 w95]
    tunnel: [w75 w94] -> w30
    tunnel: [w73 w88] -> w29
    frame False {
      n6 = call <vilib>:"DB Tools Select Data.vi"("condition"="where SNAME='D4'", "error in (no error)"=w76, "columns"=string[] ["AST", "AE", "BST", "BE", "CST", "CE", "DST", "DE"], "table"="SHIFT_TRAS", "connection reference"=w77) -> ("error out"=w83:errorcluster, "data"=w87:variant[][], "connection reference out"=w75:T14)  [unwired: 1 in]
      n7 = Variant To Data(error in=w83, type=string[][] [], Variant=w87) -> (data=w80:string[][], error out=w73:errorcluster)
      n8 = Index Array(array=w80) -> (element=w79:string[])  [unwired: 2 in]
      "SHIFT_DATA 2" <- w79
      n9 = Get Date/Time In Seconds() -> (seconds since 1Jan1904=w82:timestamp)
      n10 = call "String To Time_4.vi"("String Array In"=w79) -> ("Time Stamp Out"=w78:timestamp[])  [unwired: 9 in, 1 out]
      n11 = call "Shift Calculation_4.vi"("Current Time"=w82, "Time Stamp Out"=w78) -> ("Shift"=w74:i32)  [unwired: 8 in, 1 out]
    }
    frame True {
      n12 = call <vilib>:"DB Tools Select Data.vi"("condition"="where SNAME='D3'", "error in (no error)"=w95, "columns"=string[] ["AST", "AE", "BST", "BE", "CST", "CE"], "table"="SHIFT_TRAS", "connection reference"=w96) -> ("error out"=w100:errorcluster, "data"=w104:variant[][], "connection reference out"=w94:T14)  [unwired: 1 in]
      n13 = Variant To Data(error in=w100, type=string[][] [], Variant=w104) -> (data=w92:string[][], error out=w90:errorcluster)
      "appended array" <- w92
      n14 = Index Array(array=w92) -> (element=w91:string[])  [unwired: 2 in]
      "SHIFT_DATA" <- w91
      n15 = call "String To Time.vi"("error in (no error)"=w90, "String Array In"=w91) -> ("error out"=w89:errorcluster, "Time Stamp Out"=w97:timestamp[])  [unwired: 8 in]
      n16 = Get Date/Time In Seconds() -> (seconds since 1Jan1904=w99:timestamp)
      n17 = call "Shift Calculation.vi"("error in (no error)"=w89, "Current Time"=w99, "Time Stamp Out"=w97) -> ("error out"=w88:errorcluster, "Shift"=w98:i32)  [unwired: 7 in]
    }
  }
  n18 = control-ref of="This VI"() -> (w45:refnum<vi>)
  n19 = invoke class="VI" method="Default Vals.Reinit All"(reference=w45, error in=errorcluster {"status"=FALSE, "code"=0, "source"=""} ("error in (no error)")) -> (reference out=w44:refnum<vi>, error out=w2:errorcluster)  [unwired: 1 in, 1 out]
  n20 = case shown="3" w65 {
    tunnel: ["A" "B" "C" "D"] -> w58
    frame 1, Default {
    }
    frame 2 {
    }
    frame 3 {
    }
    frame 4 {
    }
  }
  n21 = local write "SHIFT"(w58) -> ()
  n22 = flat-sequence {
    tunnel: [w110] -> w3
    tunnel: w2 -> [w110]
    frame #0 {
      n23 = global write "DATA LOG.vi" "Auto Cycle On"(TRUE) -> ()
    }
  }
  n24 = global read "Global 1.vi" "BARCODE RECIPE"() -> (w11:string)
  n25 = call <vilib>:"DB Tools Select Data.vi"("error in (no error)"=w29, "columns"=string[] ["BARCODE_TRAC"], "table"="TRACEABILITY", "connection reference"=w30) -> ("error out"=w39:errorcluster, "data"=w38:variant[][], "connection reference out"=w17:T14)  [unwired: 2 in]
  n26 = call "PADMINI_varient_to_data.vi"("error in (no error)"=w39, "data"=w38) -> ("error out"=w15:errorcluster, "Array"=w37:string[][])  [unwired: 8 in]
  n27 = Index Array(array=w37, index (row)=0 ("disabled index (col)")) -> (element=w36:string[])  [unwired: 1 in]
  n28 = Format Into String(format string="where BARCODE_RECIPE='%s' ", w11) -> (resulting string=w9:string)  [unwired: 2 in, 1 out]
  n29 = Index Array(array=w36) -> (element=w32:string)  [unwired: 1 in]
  n30 = call <vilib>:"DB Tools Select Data.vi"("condition"=w9, "error in (no error)"=w15, "columns"=string[] ["BARCODE_RECIPE", "RECIPE_NAME"], "table"="BARCODE_RECIPE", "connection reference"=w17) -> ("error out"=w19:errorcluster, "data"=w18:variant[][], "connection reference out"=w16:T14)  [unwired: 1 in]
  n31 = To Upper Case(1:w32) -> (0:w31:string)
  n32 = Variant To Data(error in=w19, type=string[][] [], Variant=w18) -> (data=w12:string[][], error out=w14:errorcluster)
  n33 = case shown="\"False\", Default" w31 {
    tunnel: [FALSE ("BARCODE TRACEABILITY") TRUE ("BARCODE TRACEABILITY")] -> _
    tunnel: [0 1] -> w27
    frame "False", Default {
    }
    frame "TRUE" {
    }
  }
  n34 = Index Array(array=w12, index (col)=1 ("disabled index (col)")) -> (element=w7:string[])  [unwired: 1 in]
  n35 = Close Reference(reference=w44, error in (no error)=w3) -> (error out=w42:errorcluster)
  n36 = Index Array(array=w7) -> ()  [unwired: 1 in, 1 out]
  n37 = call "PADMINI_AUTO_TRACEABILITY_BYPASS.vi"("Enum"=enum16{"Read", "Write"}."Write", "error in (no error)"=w14, "I/P"=w27) -> ("error out"=w25:errorcluster)  [unwired: 7 in, 1 out]
  n38 = Obtain Queue(element data type=cluster{"CASE 2":T13} {"CASE 2"=enum."-1"}, error in (no error)=w42) -> (queue out=w70:refnum<queue>, error out=w22:errorcluster)  [unwired: 3 in, 1 out]
  n39 = flat-sequence {
    tunnel: w25 -> [w119]
    tunnel: [w119] -> w24
    frame #0 {
      w115 = FALSE
      n40 = global write "DATA LOG.vi" "OP30 ST 2 STRING"("" ("OP30 ST 2 STRING")) -> ()
      n41 = global write "DATA LOG.vi" "ST 3 STRING 2"("" ("ST 3 STRING 2")) -> ()
      n42 = global write "DATA LOG.vi" "ST 4 STRING 3"("" ("ST 4 STRING 3")) -> ()
      n43 = global write "DATA LOG.vi" "OP 100 reset"(w115) -> ()
      n44 = global write "DATA LOG.vi" "OP 110 reset"(w115) -> ()
      n45 = global write "DATA LOG.vi" "OP 30 reset"(w115) -> ()
      n46 = global write "DATA LOG.vi" "OP 20 Outputs"(w115) -> ()
      n47 = global write "DATA LOG.vi" "OP 50 reset"(w115) -> ()
      n48 = global write "DATA LOG.vi" "OP 70 reset"(w115) -> ()
      n49 = global write "DATA LOG.vi" "OP 80 reset"(w115) -> ()
      n50 = global write "DATA LOG.vi" "OP 90 reset"(w115) -> ()
      n51 = global write "DATA LOG.vi" "OP 10 Outputs"(w115) -> ()
      n52 = global write "DATA LOG.vi" "OP 30 Outputs"(w115) -> ()
      n53 = global write "DATA LOG.vi" "OP 20 reset"(w115) -> ()
      n54 = global write "DATA LOG.vi" "OP 40 reset"(w115) -> ()
      n55 = global write "DATA LOG.vi" "OP 60 reset"(w115) -> ()
      n56 = global write "DATA LOG.vi" "op 60"(0 ("op 30")) -> ()
      n57 = global write "DATA LOG.vi" "op 30"(0 ("op 30")) -> ()
      n58 = global write "DATA LOG.vi" "op 40"(0 ("op 30")) -> ()
    }
  }
  n59 = while {
    tunnel: w70 -> [w154]
    tunnel: w22 -> [w150]
    tunnel: w24 -> [w149]
    tunnel: w16 -> [w148]
    tunnel: [w123] -> w68
    tunnel: [w147] -> w67
    tunnel: FALSE -> [w146]
    tunnel: "REPORT" -> [w145]
    shift-right: [w143] -> _
    shift-left: string[] [] -> [w144]
    shift-right: [w142] -> _
    shift-left: "" ("trimmed string") -> [w141]
    shift-right: [w130] -> _
    shift-left: w1 -> [w139]
    stop <- w151 stop-if-true
    n60 = Dequeue Element(queue=w154, timeout in ms (-1)=250, error in (no error)=w150) -> (queue out=w126:refnum<queue>, element=w152:cluster{"CASE 2":T13}, error out=w153:errorcluster)  [unwired: 1 out]
    n61 = case shown="No Error" w153 {
      tunnel: w152 -> [w170 _]
      tunnel: [w166 TRUE] -> w151
      tunnel: w149 -> [w167 w1406]
      tunnel: w148 -> [w168 w1405]
      tunnel: [w164 w1406] -> w124
      tunnel: [w165 w1405] -> w147
      tunnel: w146 -> [w163 _]
      tunnel: w145 -> [w162 _]
      tunnel: w144 -> [w161 w1404]
      tunnel: [w160 w1404] -> w143
      tunnel: [w159 w1403] -> w142
      tunnel: w141 -> [w158 w1403]
      tunnel: w139 -> [w157 w1402]
      tunnel: [w156 w1402] -> w130
      tunnel: w126 -> [w155 _]
      frame No Error {
        n62 = Unbundle By Name(w170) -> ("CASE 2"=w169:T13)
        n63 = case shown="\"DATALOG4\"" w169 {
          tunnel: w168 -> [w239 w263 w331 w401 w454 w515 w569 w618 w667 w724 w773 w828 w877 w943 w989 w1036 w1085 w1133 w1182 w1231 w1271 w1330 w1389 w1397]
          tunnel: w167 -> [w236 w259 w308 w400 w441 w514 w555 w617 w653 w723 w760 w827 w863 w942 w978 w1035 w1072 w1132 w1168 w1230 w1270 w1312 w1388 w1399]
          tunnel: [FALSE FALSE FALSE FALSE FALSE FALSE FALSE FALSE FALSE FALSE FALSE FALSE FALSE FALSE FALSE FALSE FALSE FALSE FALSE FALSE FALSE FALSE FALSE TRUE] -> w166
          tunnel: [w239 w261 w328 w398 w451 w512 w566 w615 w664 w721 w770 w825 w874 w940 w986 w1033 w1083 w1130 w1179 w1228 w1268 w1327 w1389 w1396] -> w165
          tunnel: [w174 w241 w327 w395 w436 w509 w550 w612 w648 w718 w755 w822 w858 w937 w973 w1030 w1067 w1127 w1163 w1225 w1265 w1311 w1388 w1398] -> w164
          tunnel: w163 -> [_ w256 w330 w397 w453 w511 w568 w614 w666 w720 w772 w824 w876 w939 w988 w1032 w1066 w1129 w1181 w1227 w1267 w1329 _ _]
          tunnel: w162 -> [_ w262 w329 w399 w452 w513 w567 w616 w665 w722 w771 w826 w875 w941 w987 w1034 w1084 w1131 w1180 w1229 w1269 w1328 _ _]
          tunnel: w161 -> [w238 w260 w324 w392 w450 w507 w565 w610 w663 w716 w769 w820 w873 w935 w985 w1028 w1082 w1125 w1178 w1223 w1263 w1326 w1386 w1400]
          tunnel: [w238 w260 w324 w392 w450 w507 w565 w610 w663 w716 w769 w820 w873 w935 w985 w1028 w1082 w1125 w1178 w1223 w1263 w1326 w1386 w1400] -> w160
          tunnel: [w237 w255 w320 w393 w446 w506 w561 w609 w659 w715 w765 w819 w869 w934 w983 w1027 w1078 w1124 w1174 w1222 w1262 w1322 w1385 w1391] -> w159
          tunnel: w158 -> [w237 w255 w320 w393 w446 w506 w561 w609 w659 w715 w765 w819 w869 w934 w983 w1027 w1078 w1124 w1174 w1222 w1262 w1322 w1385 w1391]
          tunnel: w157 -> [w235 w249 w318 w391 w435 w505 w559 w608 w657 w714 w754 w818 w867 w933 w982 w1026 w1076 w1123 w1172 w1221 w1261 w1320 w1384 w1390]
          tunnel: [w178 w249 w318 w391 w435 w505 w559 w608 w657 w714 w754 w818 w867 w933 w982 w1026 w1076 w1123 w1172 w1221 w1261 w1320 w1384 w1390] -> w156
          tunnel: w155 -> [_ w243 _ _ _ _ _ _ _ _ _ _ _ _ _ _ _ _ _ _ _ _ _ _]
          frame "-1", Default {
            n64 = control-ref of="Final Result"() -> (w226:refnum<vi>)
            n65 = control-ref of="Top Result"() -> (w230:refnum<vi>)
            n66 = control-ref of="Bottom Result"() -> (w232:refnum<vi>)
            n67 = control-ref of="Camera Status"() -> (w231:refnum<vi>)
            n68 = control-ref of="Camera Status"() -> (w229:refnum<vi>)
            n69 = control-ref of="Final Result"() -> (w228:refnum<vi>)
            n70 = control-ref of="Final Result"() -> (w222:refnum<vi>)
            n71 = control-ref of="Shaft Status"() -> (w223:refnum<vi>)
            n72 = call "OP10 Indicators.vi"("error in (no error)"=w236, "OUTPUT INDICATOR"=w235, "Boolean in"=w226) -> ("error out"=w225:errorcluster, "OUTPUT INDICATOR"=w234:T11)  [unwired: 7 in]
            n73 = Build Array(w232, w231, w230, w229, w228) -> (w227:refnum<vi>[])
            n74 = control-ref of="RH Status"() -> (w218:refnum<vi>)
            n75 = control-ref of="Final Result"() -> (w172:refnum<vi>)
            n76 = Build Array(w223, w222) -> (w221:refnum<vi>[])
            n77 = control-ref of="LH Status"() -> (w217:refnum<vi>)
            n78 = control-ref of="Camera Status"() -> (w171:refnum<vi>)
            n79 = call "OP20 Indicators.vi"("error in (no error)"=w225, "Array"=w227, "OUTPUT INDICATOR"=w234) -> ("error out"=w224:errorcluster, "OUTPUT INDICATOR"=w233:T11)  [unwired: 7 in]
            n80 = control-ref of="Nut Status"() -> (w213:refnum<vi>)
            n81 = control-ref of="RH Status"() -> (w212:refnum<vi>)
            n82 = control-ref of="LH Status"() -> (w211:refnum<vi>)
            n83 = control-ref of="Camera Status"() -> (w210:refnum<vi>)
            n84 = control-ref of="Final Result"() -> (w209:refnum<vi>)
            n85 = Build Array(w218, w217, w171, w172) -> (w216:refnum<vi>[])
            n86 = call "OP30 Indicators.vi"("error in (no error)"=w224, "Array"=w221, "OUTPUT INDICATOR"=w233) -> ("error out"=w219:errorcluster, "OUTPUT INDICATOR"=w220:T11)  [unwired: 7 in]
            n87 = Build Array(w213, w212, w211, w210, w209) -> (w208:refnum<vi>[])
            n88 = call "OP40 Indicators.vi"("error in (no error)"=w219, "Array"=w216, "OUTPUT INDICATOR"=w220) -> ("error out"=w215:errorcluster, "OUTPUT INDICATOR"=w214:T11)  [unwired: 7 in]
            n89 = control-ref of="Screw 1 Status"() -> (w204:refnum<vi>)
            n90 = control-ref of="Screw 2 Status"() -> (w203:refnum<vi>)
            n91 = control-ref of="Screw 3 Status"() -> (w202:refnum<vi>)
            n92 = control-ref of="Screw 4 Status"() -> (w201:refnum<vi>)
            n93 = control-ref of="Screw 5 Status"() -> (w200:refnum<vi>)
            n94 = control-ref of="Screw 6 Status"() -> (w199:refnum<vi>)
            n95 = control-ref of="Final Result"() -> (w198:refnum<vi>)
            n96 = control-ref of="Final Result"() -> (w195:refnum<vi>)
            n97 = call "OP50 Indicators.vi"("error in (no error)"=w215, "Array"=w208, "OUTPUT INDICATOR"=w214) -> ("error out"=w207:errorcluster, "OUTPUT INDICATOR"=w206:T11)  [unwired: 7 in]
            n98 = Build Array(w204, w203, w202, w201, w200, w199, w198) -> (w205:refnum<vi>[])
            n99 = control-ref of="Loctite Status"() -> (w191:refnum<vi>)
            n100 = control-ref of="Final Result"() -> (w190:refnum<vi>)
            n101 = Build Array(w195) -> (w194:refnum<vi>[])
            n102 = call "OP60 Indicators.vi"("error in (no error)"=w207, "Array"=w205, "OUTPUT INDICATOR"=w206) -> ("error out"=w197:errorcluster, "OUTPUT INDICATOR"=w196:T11)  [unwired: 7 in]
            n103 = call "OP70 Indicators.vi"("error in (no error)"=w197, "Array"=w194, "OUTPUT INDICATOR"=w196) -> ("error out"=w193:errorcluster, "OUTPUT INDICATOR"=w192:T11)  [unwired: 7 in]
            n104 = control-ref of="Seat Status"() -> (w186:refnum<vi>)
            n105 = control-ref of="Final Result"() -> (w185:refnum<vi>)
            n106 = control-ref of="Final Result"() -> (w181:refnum<vi>)
            n107 = control-ref of="Camera Status"() -> (w173:refnum<vi>)
            n108 = Build Array(w191, w190) -> (w189:refnum<vi>[])
            n109 = call "OP80 Indicators.vi"("error in (no error)"=w193, "Array"=w189, "OUTPUT INDICATOR"=w192) -> ("error out"=w187:errorcluster, "OUTPUT INDICATOR"=w188:T11)  [unwired: 7 in]
            n110 = Build Array(w186, w185) -> (w184:refnum<vi>[])
            n111 = Build Array(w181, w173) -> (w180:refnum<vi>[])
            n112 = call "OP90 Indicators.vi"("error in (no error)"=w187, "Array"=w184, "OUTPUT INDICATOR"=w188) -> ("error out"=w183:errorcluster, "OUTPUT INDICATOR"=w182:T11)  [unwired: 7 in]
            n113 = call "OP100 Indicators.vi"("error in (no error)"=w183, "Array"=w180, "OUTPUT INDICATOR"=w182) -> ("error out"=w174:errorcluster, "OUTPUT INDICATOR"=w179:T11)  [unwired: 7 in]
            n114 = call "PADMINI_AUTO_BARCODE_STRING 110.vi"("Enum"=enum16{"Read", "Write"}."Read", "error in (no error)"=w174) -> ("Input 2"=w176:string[])  [unwired: 8 in, 1 out]
            n115 = Index Array(array=w176) -> (element=w177:string)  [unwired: 1 in]
            n116 = Bundle By Name(cluster=w179, "OP - 110.BARCODE"=w177) -> (w178:T11)
          }
          frame "SCAN1" {
            # "STATION OP 10"
            n117 = global read "Global 1.vi" "BARCODE RECIPE"() -> (w250:string)
            n118 = call "PADMINI_AUTO_BARCODE_STRING.vi"("Enum"=enum16{"Read", "Write"}."Read", "error in (no error)"=w259) -> ("error out"=w258:errorcluster, "Input 2"=w246:string[])  [unwired: 8 in]
            n119 = Index Array(array=w246) -> (element=w245:string)  [unwired: 1 in]
            n120 = call <vilib>:"Trim Whitespace.vi"("string"=w245) -> ("trimmed string"=w244:string)  [unwired: 1 in]
            n121 = Match Pattern(string=w244, regular expression=w250) -> (match substring=w253:string)  [unwired: 1 in, 3 out]
            n122 = String Length(string=w250) -> (length=w252:i32)
            n123 = String Length(string=w253) -> (length=w251:i32)
            n124 = Equal?(x=w252, y=w251) -> (x = y?=w257:bool)
            n125 = case shown="False" w256 {
              tunnel: w263 -> [w289 w307]
              tunnel: w258 -> [w288 w305]
              tunnel: w262 -> [w287 _]
              tunnel: [w286 w304] -> w248
              tunnel: [w285 w307] -> w261
              tunnel: w257 -> [_ _]
              tunnel: w244 -> [w284 _]
              tunnel: [w283 TRUE] -> w242
              frame False {
                n126 = Format Into String(format string="where BARCODE='%s'", w284) -> (resulting string=w280:string)  [unwired: 2 in, 1 out]
                n127 = call <vilib>:"DB Tools Select Data.vi"("condition"=w280, "error in (no error)"=w288, "columns"=string[] ["BARCODE", "OP10_FINAL_RESULT"], "table"=w287, "connection reference"=w289) -> ("error out"=w279:errorcluster, "data"=w278:variant[][], "connection reference out"=w285:T14)  [unwired: 1 in]
                n128 = call "PADMINI_varient_to_data.vi"("error in (no error)"=w279, "data"=w278) -> ("error out"=w276:errorcluster, "Array"=w272:string[][])  [unwired: 8 in]
                n129 = Index Array(array=w272, index (row)=0) -> (element=→"SCAN OP10":string[])  [unwired: 1 in]
                n130 = Index Array(array=w272, index (row)=0, index (col)=1 ("index (row)")) -> (element=w273:string)
                n131 = Empty Array?(array=w272) -> (empty?=w277:bool)
                n132 = case shown="False" w277 {
                  tunnel: w276 -> [w299 w301]
                  tunnel: [w298 w301] -> w286
                  tunnel: [FALSE TRUE] -> w283
                  tunnel: w273 -> [w293 _]
                  frame False {
                    w292 = "OK"  # y
                    w295 = i32[] [1, 0]  # I/P
                    w294 = i32[] [0, 1]  # I/P
                    # "OP10 CURRENT STATION OK-NG\nPART REPEAT"
                    n133 = Equal?(x=w293, y=w292) -> (x = y?=w291:bool)
                    n134 = Select(t=w295, s=w291, f=w294) -> (s? t:f=w290:i32[])
                    "OP10 STATUS" <- w290
                    n135 = call "PADMINI_AUTO_BARCODE_STATUS.vi"("Enum"=enum16{"Read", "Write"}."Write", "error in (no error)"=w299, "I/P"=w290) -> ("error out"=w298:errorcluster)  [unwired: 7 in, 1 out]
                  }
                  frame True {
                    # "OP10 NEW part"
                  }
                }
              }
              frame True {
                w303 = i32[] [0, 1]  # I/P
                n136 = call "PADMINI_AUTO_BARCODE_STATUS.vi"("Enum"=enum16{"Read", "Write"}."Write", "error in (no error)"=w305, "I/P"=w303) -> ("error out"=w304:errorcluster)  [unwired: 7 in, 1 out]
              }
            }
            n137 = flat-sequence {
              tunnel: [w269] -> w247
              tunnel: w248 -> [w269]
              frame #0 {
                # "UPDATE op 10 sCAN sTATUS"
                n138 = global write "DATA LOG.vi" "OP 10 Outputs"(TRUE) -> ()
              }
            }
            n139 = call <vilib>:"Clear Errors.vi"("error in (no error)"=w247) -> ("error out"=w241:errorcluster)  [unwired: 5 in, 1 out]
            n140 = case shown="True" w242 {
              tunnel: w243 -> [_ w267]
              tunnel: w241 -> [_ w265]
              frame False {
              }
              frame True {
                w266 = cluster{"CASE 2":T13} {"CASE 2"=enum."DATALOG1"}  # element
                n141 = Enqueue Element(queue=w267, element=w266, error in (no error)=w265) -> ()  [unwired: 1 in, 3 out]
              }
            }
          }
          frame "DATALOG1" {
            w322 = T15 2 items=["no dialog", "OK message", "continue or stop message", "OK message + warnings", "continue/stop + warnings"] ("type of dialog (OK msg:1)")
            # "cycle result status\nwhether it was ok or nok\nor abortted in between"
            # "Printed QR Code data string"
            # "datalog of OP 10"
            n142 = call "PADMINI_AUTO_BARCODE_STRING.vi"("Enum"=enum16{"Read", "Write"}."Read", "error in (no error)"=w308) -> ("Input 2"=w315:string[])  [unwired: 8 in, 1 out]
            n143 = call "PADMINI_AUTO_CYCLE VALUE 10.vi"("Enum"=enum16{"Read", "Write"}."Read", "error in (no error)"=w308) -> ("error out"=w311:errorcluster, "Input 2"=w310:sgl[])  [unwired: 8 in]
            n144 = Index Array(array=w310) -> (element=w309:sgl)  [unwired: 1 in]
            n145 = Index Array(array=w315) -> (element #1=w314:string, element #2=w313:string)  [unwired: 2 in]
            n146 = Number To Fractional String(number=w309, precision (6)=i16 2) -> (F-format string=w316:string)  [unwired: 2 in]
            n147 = call <vilib>:"Trim Whitespace.vi"("string"=w314) -> ("trimmed string"=w325:string)  [unwired: 1 in]
            n148 = case shown="False" w330 {
              tunnel: w331 -> [w355 w390]
              tunnel: w311 -> [w357 w389]
              tunnel: [w363 w388] -> w328
              tunnel: [w362 w387] -> w323
              tunnel: w329 -> [w352 _]
              tunnel: w325 -> [w349 _]
              tunnel: w313 -> [w359 w380]
              tunnel: w316 -> [w343 w379]
              frame False {
                w351 = string[] ["BARCODE", "SHIFT", "OP10_DATE", "OP10_LEAK_RATE_SCCM", "OP10_FINAL_RESULT"]
                # "ST1 RESULT"
                # "DO TRACEBILITY"
                n149 = local read "SHIFT"() -> (w361:string)
                n150 = Format Into String(format string="Where BARCODE='%s' ", w349) -> (resulting string=w344:string)  [unwired: 2 in, 1 out]
                n151 = call <vilib>:"DB Tools Select Data.vi"("condition"=w344, "error in (no error)"=w357, "columns"=w351, "table"=w352, "connection reference"=w355) -> ("error out"=w353:errorcluster, "data"=w356:variant[][], "connection reference out"=w354:T14)  [unwired: 1 in]
                n152 = call "PADMINI_SHIFT_DATE.vi"("SHIFT"=w361) -> ("date/time string"=w360:string)  [unwired: 10 in]
                n153 = Variant To Data(error in=w353, type=string[][] [], Variant=w356) -> (data=w347:string[][], error out=w345:errorcluster)
                n154 = Bundle("trimmed string"=w349, "SHIFT"=w361, "date/time string"=w360, w343, "Input 2"=w359) -> (w358:T16)  [unwired: 1 in]
                n155 = Empty Array?(array=w347) -> (empty?=w346:bool)
                n156 = case shown="False" w346 {
                  tunnel: w354 -> [w368 w378]
                  tunnel: w345 -> [w367 w377]
                  tunnel: [w371 w376] -> w363
                  tunnel: [w370 w375] -> w362
                  tunnel: w351 -> [w365 w374]
                  tunnel: w352 -> [w366 w373]
                  tunnel: w358 -> [w369 w372]
                  tunnel: w344 -> [w364 _]
                  frame False {
                    n157 = call <vilib>:"DB Tools Update Data.vi"("condition"=w364, "data"=w369, "error in (no error)"=w367, "columns"=w365, "table"=w366, "connection reference"=w368) -> ("error out"=w370:errorcluster, "connection reference out"=w371:T14)  [unwired: 4 in]
                  }
                  frame True {
                    n158 = call <vilib>:"DB Tools Insert Data.vi"("data"=w372, "error in (no error)"=w377, "columns"=w374, "table"=w373, "connection reference"=w378) -> ("error out"=w375:errorcluster, "connection reference out"=w376:T14)  [unwired: 5 in]
                  }
                }
              }
              frame True {
                # "Trac BYPASS"
                n159 = local read "SHIFT"() -> (w385:string)
                n160 = call "PADMINI_SHIFT_DATE.vi"("SHIFT"=w385) -> ("date/time string"=w384:string)  [unwired: 10 in]
                n161 = Bundle("SHIFT"=w385, "date/time string"=w384, "Input 2"=w380, w379) -> (w383:T17)  [unwired: 1 in]
                n162 = To Variant(anything=w383) -> (Variant=w382:variant)
                n163 = call <vilib>:"DB Tools Insert Data.vi"("data"=w382, "error in (no error)"=w389, "columns"=string[] ["DATE", "SHIFT", "OP10_LEAK_RAT", "OP10_FINAL_RST"], "table"="ST1_REPORT", "connection reference"=w390) -> ("error out"=w387:errorcluster, "connection reference out"=w388:T14)  [unwired: 5 in]
              }
            }
            n164 = call <vilib>:"Simple Error Handler.vi"("type of dialog (OK msg:1)"=w322, "error in (no error)"=w323) -> ("error out"=w321:errorcluster)  [unwired: 3 in, 4 out]
            n165 = call <vilib>:"Clear Errors.vi"("error in (no error)"=w321) -> ("error out"=w319:errorcluster)  [unwired: 5 in, 1 out]
            n166 = disable-structure shown="Enabled" {
              disable-tunnel: [w341 w342] -> w327
              disable-tunnel: w319 -> [w340 w342]
              frame Disabled {
                w335 = refnum<vi> refnum  # Boolean
                n167 = property on="OP - 10" class="Clust"(error in=w340) -> (error out=w334:errorcluster, "Controls[]"=w338:refnum<vi>[])  [unwired: 1 in, 1 out]
                n168 = Index Array(array=w338, index=2) -> (element=w336:refnum<vi>)
                n169 = To More Specific Class(target class=w335, reference=w336, error in=w334) -> (specific class reference=w339:refnum<vi>, error out=w333:errorcluster)
                n170 = call "PADMINI_BOOL_COLOR_CHANGE.vi"("error in (no error)"=w333, "Boolean in"=w339) -> ("error out"=w341:errorcluster)  [unwired: 9 in]
              }
              frame Enabled {
              }
            }
          }
          frame "SCAN2" {
            # "Barcode Status\n0-Ideal, 1-Ok, 2-Nok, 3-Prev Station Not Done,\n4-Prev Station Nok,\n5- Already Done"
            # "STATION OP 20"
            n171 = case shown="False" w397 {
              tunnel: w401 -> [w426 w432]
              tunnel: w400 -> [w419 w430]
              tunnel: w399 -> [w407 _]
              tunnel: [w421 w429] -> w396
              tunnel: [w420 w432] -> w398
              tunnel: [w408 "" ("trimmed string")] -> _
              frame False {
                # "ST2 RESULT"
                # "ST1 RESULT"
                # "2 FOR EMPTY BARCODE READ OR MISMATCH"
                n172 = call "PADMINI_AUTO_BARCODE_STRING2.vi"("Enum"=enum16{"Read", "Write"}."Read", "error in (no error)"=w419) -> ("error out"=w418:errorcluster, "Input 2"=w410:string[])  [unwired: 8 in]
                n173 = global read "Global 1.vi" "BARCODE RECIPE"() -> (w411:string)
                n174 = Index Array(array=w410) -> (element=w409:string)  [unwired: 1 in]
                n175 = call <vilib>:"Trim Whitespace.vi"("string"=w409) -> ("trimmed string"=w408:string)  [unwired: 1 in]
                n176 = Match Pattern(string=w408, regular expression=w411) -> (match substring=w412:string)  [unwired: 1 in, 3 out]
                n177 = String Length(string=w411) -> (length=w414:i32)
                n178 = String Length(string=w412) -> (length=w413:i32)
                n179 = Format Into String(format string="WHERE BARCODE  ='%s'", w408) -> (resulting string=w415:string)  [unwired: 2 in, 1 out]
                n180 = Equal?(x=w414, y=w413) -> ()  [unwired: 1 out]
                n181 = call <vilib>:"DB Tools Select Data.vi"("condition"=w415, "error in (no error)"=w418, "columns"=string[] ["BARCODE", "OP10_FINAL_RESULT", "OP20_FINAL_RESULT"], "table"=w407, "connection reference"=w426) -> ("error out"=w424:errorcluster, "data"=w423:variant[][], "connection reference out"=w420:T14)  [unwired: 1 in]
                n182 = call "PADMINI_varient_to_data.vi"("error in (no error)"=w424, "data"=w423) -> ("error out"=w422:errorcluster, "Array"=w404:string[][])  [unwired: 8 in]
                n183 = Index Array(array=w404, index (row)=0 ("disabled index (col)")) -> (element=→"SCAN OP20":string[])  [unwired: 1 in]
                n184 = call "RESPONSE_LOGIC.vi"("Array"=w404) -> ("Not Found"=w402:i32[])  [unwired: 10 in]
                "OP20 STATUS" <- w402
                n185 = call "PADMINI_AUTO_BARCODE_STATUS 20.vi"("Enum"=enum16{"Read", "Write"}."Write", "error in (no error)"=w422, "I/P"=w402) -> ("error out"=w421:errorcluster)  [unwired: 7 in, 1 out]
              }
              frame True {
                w427 = i32[] [0, 0, 0, 0, 0]  # I/P
                n186 = call "PADMINI_AUTO_BARCODE_STATUS 20.vi"("Enum"=enum16{"Read", "Write"}."Write", "error in (no error)"=w430, "I/P"=w427) -> ("error out"=w429:errorcluster)  [unwired: 7 in, 1 out]
              }
            }
            n187 = flat-sequence {
              tunnel: [w434] -> w395
              tunnel: w396 -> [w434]
              frame #0 {
                # "UPDATE op 20 SCAN sTATUS"
                n188 = global write "DATA LOG.vi" "OP 20 Outputs"(TRUE) -> ()
              }
            }
          }
          frame "DATALOG2" {
            (unwired) string[] ["OP20_DATE", "OP20_LOWER_BEARING_DIS", "OP20_LOWER_BEARING_LOAD", "OP20_UPPER_BEARING_DIS", "OP20_UPPER_BEARING_LOAD", "OP20_LOWER_BEARING_RST", "OP20_BOTTOM_CAMERA_STATUS", "OP20_UPPER_SIM_STATUS", "OP20_UPPER_BERAING_RST", "OP20_UPPER_CAMERA_STATUS", "OP20_FINAL_RST"]
            w448 = T15 2 items=["no dialog", "OK message", "continue or stop message", "OK message + warnings", "continue/stop + warnings"] ("type of dialog (OK msg:1)")
            # "Printed QR Code data string"
            # "datalog of OP 20"
            n189 = call "PADMINI_AUTO_BARCODE_STRING2.vi"("Enum"=enum16{"Read", "Write"}."Read", "error in (no error)"=w441) -> ("error out"=w443:errorcluster, "Input 2"=w437:string[])  [unwired: 8 in]
            n190 = call "PADMINI_AUTO_CYCLE VALUE 20.vi"("Enum"=enum16{"Read", "Write"}."Read", "error in (no error)"=w441) -> ("Input 2"=w439:sgl[])  [unwired: 8 in, 1 out]
            n191 = Number To Fractional String(number=w439, precision (6)=i16 2) -> (F-format string=w438:string[])  [unwired: 2 in]
            n192 = case shown="False" w453 {
              tunnel: w454 -> [w478 w504]
              tunnel: w443 -> [w479 w503]
              tunnel: [w482 w502] -> w451
              tunnel: [w481 w501] -> w449
              tunnel: w452 -> [w477 _]
              tunnel: w438 -> [w474 w486]
              tunnel: w437 -> [w468 w487]
              frame False {
                # "ST2 RESULT"
                # "DO TRACEBILITY"
                n193 = Index Array(array=w468) -> (element #1=w469:string, element #2=w464:string, element #3=w463:string, element #4=w462:string, element #5=w461:string, element #6=w460:string, element #7=w459:string)  [unwired: 7 in]
                n194 = local read "SHIFT"() -> (w480:string)
                n195 = Index Array(array=w474) -> (element #1=w473:string, element #2=w472:string, element #3=w466:string, element #4=w465:string)  [unwired: 4 in]
                n196 = call <vilib>:"Trim Whitespace.vi"("string"=w469) -> ("trimmed string"=w470:string)  [unwired: 1 in]
                n197 = call "PADMINI_SHIFT_DATE.vi"("SHIFT"=w480) -> ("date/time string"=w467:string)  [unwired: 10 in]
                n198 = Format Into String(format string="Where BARCODE='%s' ", w470) -> (resulting string=w475:string)  [unwired: 2 in, 1 out]
                n199 = Bundle("date/time string"=w467, "Input 2"=w473, "Input 2"=w472, "Input 2"=w466, "Input 2"=w465, "Input 2"=w464, "Input 2"=w463, "Input 2"=w462, "Input 2"=w461, "Input 2"=w460, "Input 2"=w459) -> (w471:T18)  [unwired: 1 in]
                n200 = call <vilib>:"DB Tools Update Data.vi"("condition"=w475, "data"=w471, "error in (no error)"=w479, "columns"=string[] ["OP20_DATE", "OP20_BOTTOM_DISPLACE_mm", "OP20_BOTTOM_LOAD_kg", "OP20_TOP_DISPLACE_mm", "OP20_TOP_LOAD_kg", "OP20_BOTTOM_RESULT", "OP20_BOTTOM_CAMERA_STATUS", "OP20_TOP_SIM_STATUS", "OP20_TOP_RESULT", "OP20_TOP_CAMERA_STATUS", "OP20_FINAL_RESULT"], "table"=w477, "connection reference"=w478) -> ("error out"=w481:errorcluster, "connection reference out"=w482:T14)  [unwired: 4 in]
              }
              frame True {
                n201 = local read "SHIFT"() -> (w484:string)
                n202 = Index Array(array=w487) -> (element #2=w493:string, element #3=w492:string, element #4=w491:string, element #5=w490:string, element #6=w489:string, element #7=w483:string)  [unwired: 7 in, 1 out]
                n203 = call "PADMINI_SHIFT_DATE.vi"("SHIFT"=w484) -> ("date/time string"=w485:string)  [unwired: 10 in]
                n204 = Index Array(array=w486) -> (element #1=w497:string, element #2=w496:string, element #3=w495:string, element #4=w494:string)  [unwired: 4 in]
                n205 = Bundle("date/time string"=w485, "SHIFT"=w484, "Input 2"=w497, "Input 2"=w496, "Input 2"=w493, "Input 2"=w492, "Input 2"=w495, "Input 2"=w494, "Input 2"=w491, "Input 2"=w490, "Input 2"=w489, "Input 2"=w483) -> (w488:T19)  [unwired: 1 in]
                n206 = To Variant(anything=w488) -> (Variant=w499:variant)
                n207 = call <vilib>:"DB Tools Insert Data.vi"("data"=w499, "error in (no error)"=w503, "columns"=string[] ["DATE", "SHIFT", "ST2_LOWER_BEARING_DIS", "ST2_LOWER_BEARING_LOAD", "ST2_BOTTOM_CAMERA_STATUS", "ST2_LOWER_BEARING_RST", "ST2_UPPER_BEARING_DIS", "ST2_UPPER_BEARING_LOAD", "ST2_UPPER_SIM_STATUS", "ST2_UPPER_CAMERA_STATUS", "ST2_UPPER_BERAING_RST", "ST2_FINAL_RST"], "table"="ST2_REPORT", "connection reference"=w504) -> ("error out"=w501:errorcluster, "connection reference out"=w502:T14)  [unwired: 5 in]
              }
            }
            n208 = call <vilib>:"Simple Error Handler.vi"("type of dialog (OK msg:1)"=w448, "error in (no error)"=w449) -> ("error out"=w447:errorcluster)  [unwired: 3 in, 4 out]
            n209 = call <vilib>:"Clear Errors.vi"("error in (no error)"=w447) -> ("error out"=w445:errorcluster)  [unwired: 5 in, 1 out]
            n210 = flat-sequence {
              tunnel: [w457] -> w436
              tunnel: w445 -> [w457]
              frame #0 {
                # "UPDATE op 20 save"
                n211 = global write "DATA LOG.vi" "OP 20 reset"(TRUE) -> ()
              }
            }
          }
          frame "SCAN3" {
            # "STATION OP 30"
            n212 = case shown="False" w511 {
              tunnel: w515 -> [w541 w547]
              tunnel: w514 -> [w534 w545]
              tunnel: w513 -> [w521 _]
              tunnel: [w536 w544] -> w510
              tunnel: [w535 w547] -> w512
              tunnel: [w522 "" ("trimmed string")] -> _
              frame False {
                n213 = call "PADMINI_AUTO_BARCODE_STRING 30.vi"("Enum"=enum16{"Read", "Write"}."Read", "error in (no error)"=w534) -> ("error out"=w533:errorcluster, "Input 2"=w524:string[])  [unwired: 8 in]
                n214 = global read "Global 1.vi" "BARCODE RECIPE"() -> (w525:string)
                n215 = Index Array(array=w524) -> (element=w523:string)  [unwired: 1 in]
                n216 = call <vilib>:"Trim Whitespace.vi"("string"=w523) -> ("trimmed string"=w522:string)  [unwired: 1 in]
                n217 = Match Pattern(string=w522, regular expression=w525) -> (match substring=w526:string)  [unwired: 1 in, 3 out]
                n218 = String Length(string=w525) -> (length=w528:i32)
                n219 = String Length(string=w526) -> (length=w527:i32)
                n220 = Equal?(x=w522, y="") -> ()  [unwired: 1 out]
                n221 = Format Into String(format string="WHERE BARCODE  ='%s'", w522) -> (resulting string=w530:string)  [unwired: 2 in, 1 out]
                n222 = Equal?(x=w528, y=w527) -> ()  [unwired: 1 out]
                n223 = call <vilib>:"DB Tools Select Data.vi"("condition"=w530, "error in (no error)"=w533, "columns"=string[] ["BARCODE", "OP20_FINAL_RESULT", "OP30_FINAL_RESULT"], "table"=w521, "connection reference"=w541) -> ("error out"=w539:errorcluster, "data"=w538:variant[][], "connection reference out"=w535:T14)  [unwired: 1 in]
                n224 = call "PADMINI_varient_to_data.vi"("error in (no error)"=w539, "data"=w538) -> ("error out"=w537:errorcluster, "Array"=w518:string[][])  [unwired: 8 in]
                n225 = Index Array(array=w518, index (row)=0 ("disabled index (col)")) -> (element=→"SCAN OP30":string[])  [unwired: 1 in]
                n226 = call "RESPONSE_LOGIC.vi"("Array"=w518) -> ("Not Found"=w516:i32[])  [unwired: 10 in]
                "OP30 STATUS" <- w516
                n227 = call "PADMINI_AUTO_BARCODE_STATUS 30.vi"("Enum"=enum16{"Read", "Write"}."Write", "error in (no error)"=w537, "I/P"=w516) -> ("error out"=w536:errorcluster)  [unwired: 7 in, 1 out]
              }
              frame True {
                w542 = i32[] [0, 0, 0, 0, 0]  # I/P
                n228 = call "PADMINI_AUTO_BARCODE_STATUS 30.vi"("Enum"=enum16{"Read", "Write"}."Write", "error in (no error)"=w545, "I/P"=w542) -> ("error out"=w544:errorcluster)  [unwired: 7 in, 1 out]
              }
            }
            n229 = flat-sequence {
              tunnel: [w549] -> w509
              tunnel: w510 -> [w549]
              frame #0 {
                # "UPDATE op 30 SCAN sTATUS"
                n230 = global write "DATA LOG.vi" "OP 30 Outputs"(TRUE) -> ()
              }
            }
          }
          frame "DATALOG3" {
            (unwired) string[] ["OP30_DATE", "OP30_DISPLACEMENT", "OP30_SHAFT_PRESS_LOAD", "OP30_SHAFT_STATUS", "OP30_FINAL_RST"]
            w563 = T15 2 items=["no dialog", "OK message", "continue or stop message", "OK message + warnings", "continue/stop + warnings"] ("type of dialog (OK msg:1)")
            # "Printed QR Code data string"
            # "datalog of OP 30"
            n231 = call "PADMINI_AUTO_BARCODE_STRING 30.vi"("Enum"=enum16{"Read", "Write"}."Read", "error in (no error)"=w555) -> ("error out"=w557:errorcluster, "Input 2"=w551:string[])  [unwired: 8 in]
            n232 = call "PADMINI_AUTO_CYCLE VALUE 30.vi"("Enum"=enum16{"Read", "Write"}."Read", "error in (no error)"=w555) -> ("Input 2"=w553:sgl[])  [unwired: 8 in, 1 out]
            n233 = Number To Fractional String(number=w553, precision (6)=i16 2) -> (F-format string=w552:string[])  [unwired: 2 in]
            n234 = case shown="False" w568 {
              tunnel: w569 -> [w587 w607]
              tunnel: w557 -> [w588 w606]
              tunnel: [w591 w605] -> w566
              tunnel: [w590 w604] -> w564
              tunnel: w567 -> [w586 _]
              tunnel: w552 -> [w583 w592]
              tunnel: w551 -> [w577 w593]
              frame False {
                # "DO TRACEBILITY"
                n235 = Index Array(array=w577) -> (element #1=w578:string, element #2=w576:string, element #3=w575:string)  [unwired: 3 in]
                n236 = local read "SHIFT"() -> (w589:string)
                n237 = Index Array(array=w583) -> (element #1=w582:string, element #2=w581:string)  [unwired: 2 in]
                n238 = call <vilib>:"Trim Whitespace.vi"("string"=w578) -> ("trimmed string"=w579:string)  [unwired: 1 in]
                n239 = call "PADMINI_SHIFT_DATE.vi"("SHIFT"=w589) -> ("date/time string"=w574:string)  [unwired: 10 in]
                n240 = Format Into String(format string="Where BARCODE='%s' ", w579) -> (resulting string=w584:string)  [unwired: 2 in, 1 out]
                n241 = Bundle("date/time string"=w574, "Input 2"=w582, "Input 2"=w581, "Input 2"=w576, "Input 2"=w575) -> (w580:T20)  [unwired: 1 in]
                n242 = call <vilib>:"DB Tools Update Data.vi"("condition"=w584, "data"=w580, "error in (no error)"=w588, "columns"=string[] ["OP30_DATE", "OP30_DISPLACEMENT_mm", "OP30_SHAFT_PRESS_LOAD_kg", "OP30_SHAFT_STATUS", "OP30_FINAL_RESULT"], "table"=w586, "connection reference"=w587) -> ("error out"=w590:errorcluster, "connection reference out"=w591:T14)  [unwired: 4 in]
              }
              frame True {
                # "TRAC BYPASS"
                n243 = local read "SHIFT"() -> (w594:string)
                n244 = call "PADMINI_SHIFT_DATE.vi"("SHIFT"=w594) -> ("date/time string"=w595:string)  [unwired: 10 in]
                n245 = Index Array(array=w593) -> (element #2=w599:string, element #3=w598:string)  [unwired: 3 in, 1 out]
                n246 = Index Array(array=w592) -> (element #1=w601:string, element #2=w600:string)  [unwired: 2 in]
                n247 = Bundle("date/time string"=w595, "SHIFT"=w594, "Input 2"=w601, "Input 2"=w600, "Input 2"=w599, "Input 2"=w598) -> (w596:T21)  [unwired: 1 in]
                n248 = To Variant(anything=w596) -> (Variant=w597:variant)
                n249 = call <vilib>:"DB Tools Insert Data.vi"("data"=w597, "error in (no error)"=w606, "columns"=string[] ["DATE", "SHIFT", "ST3_DISPLACEMENT", "ST3_LOAD", "ST3_MIDDLE_GEAR_SHAFT_STATUS", "ST3_FINAL_RST"], "table"="ST3_REPORT", "connection reference"=w607) -> ("error out"=w604:errorcluster, "connection reference out"=w605:T14)  [unwired: 5 in]
              }
            }
            n250 = call <vilib>:"Simple Error Handler.vi"("type of dialog (OK msg:1)"=w563, "error in (no error)"=w564) -> ("error out"=w562:errorcluster)  [unwired: 3 in, 4 out]
            n251 = call <vilib>:"Clear Errors.vi"("error in (no error)"=w562) -> ("error out"=w560:errorcluster)  [unwired: 5 in, 1 out]
            n252 = flat-sequence {
              tunnel: [w572] -> w550
              tunnel: w560 -> [w572]
              frame #0 {
                # "UPDATE op 20 save"
                n253 = global write "DATA LOG.vi" "OP 30 reset"(TRUE) -> ()
              }
            }
          }
          frame "SCAN4" {
            # "STATION OP 40"
            n254 = case shown="False" w614 {
              tunnel: w618 -> [w639 w645]
              tunnel: w617 -> [w632 w644]
              tunnel: w616 -> [w624 _]
              tunnel: [w634 w643] -> w613
              tunnel: [w633 w645] -> w615
              tunnel: [w625 "" ("trimmed string")] -> _
              frame False {
                n255 = call "PADMINI_AUTO_BARCODE_STRING 40.vi"("Enum"=enum16{"Read", "Write"}."Read", "error in (no error)"=w632) -> ("error out"=w631:errorcluster, "Input 2"=w627:string[])  [unwired: 8 in]
                n256 = Index Array(array=w627) -> (element=w626:string)  [unwired: 1 in]
                n257 = call <vilib>:"Trim Whitespace.vi"("string"=w626) -> ("trimmed string"=w625:string)  [unwired: 1 in]
                n258 = Format Into String(format string="WHERE BARCODE  ='%s'", w625) -> (resulting string=w628:string)  [unwired: 2 in, 1 out]
                n259 = call <vilib>:"DB Tools Select Data.vi"("condition"=w628, "error in (no error)"=w631, "columns"=string[] ["BARCODE", "OP30_FINAL_RESULT", "OP40_FINAL_RESULT"], "table"=w624, "connection reference"=w639) -> ("error out"=w637:errorcluster, "data"=w636:variant[][], "connection reference out"=w633:T14)  [unwired: 1 in]
                n260 = call "PADMINI_varient_to_data.vi"("error in (no error)"=w637, "data"=w636) -> ("error out"=w635:errorcluster, "Array"=w621:string[][])  [unwired: 8 in]
                n261 = call "RESPONSE_LOGIC.vi"("Array"=w621) -> ("Not Found"=w619:i32[])  [unwired: 10 in]
                "OP40 STATUS" <- w619
                n262 = Index Array(array=w621, index (row)=0 ("disabled index (col)")) -> (element=→"SCAN OP40":string[])  [unwired: 1 in]
                n263 = call "PADMINI_AUTO_BARCODE_STATUS 40.vi"("Enum"=enum16{"Read", "Write"}."Write", "error in (no error)"=w635, "I/P"=w619) -> ("error out"=w634:errorcluster)  [unwired: 7 in, 1 out]
              }
              frame True {
                w640 = i32[] [0, 0, 0, 0, 0]  # I/P
                n264 = call "PADMINI_AUTO_BARCODE_STATUS 40.vi"("Enum"=enum16{"Read", "Write"}."Write", "error in (no error)"=w644, "I/P"=w640) -> ("error out"=w643:errorcluster)  [unwired: 7 in, 1 out]
              }
            }
            n265 = flat-sequence {
              tunnel: [w647] -> w612
              tunnel: w613 -> [w647]
              frame #0 {
                # "UPDATE op 40 SCAN sTATUS"
                n266 = global write "DATA LOG.vi" "OP 40 Outputs"(TRUE) -> ()
              }
            }
          }
          frame "DATALOG4" {
            w661 = T15 2 items=["no dialog", "OK message", "continue or stop message", "OK message + warnings", "continue/stop + warnings"] ("type of dialog (OK msg:1)")
            # "datalog of OP 40"
            n267 = call "PADMINI_AUTO_BARCODE_STRING 40.vi"("Enum"=enum16{"Read", "Write"}."Read", "error in (no error)"=w653) -> ("error out"=w655:errorcluster, "Input 2"=w649:string[])  [unwired: 8 in]
            n268 = call "PADMINI_AUTO_CYCLE VALUE 40.vi"("Enum"=enum16{"Read", "Write"}."Read", "error in (no error)"=w653) -> ("Input 2"=w651:sgl[])  [unwired: 8 in, 1 out]
            n269 = Number To Fractional String(number=w651, precision (6)=i16 2) -> (F-format string=w650:string[])  [unwired: 2 in]
            n270 = case shown="False" w666 {
              tunnel: w667 -> [w689 w713]
              tunnel: w655 -> [w690 w712]
              tunnel: [w693 w711] -> w664
              tunnel: [w692 w710] -> w662
              tunnel: w665 -> [w688 _]
              tunnel: w650 -> [w684 w695]
              tunnel: w649 -> [w679 w694]
              frame False {
                # "DO TRACEBILITY"
                n271 = Index Array(array=w679) -> (element #1=w680:string, element #2=w675:string, element #3=w674:string, element #4=w672:string, element #5=w671:string)  [unwired: 5 in]
                n272 = local read "SHIFT"() -> (w691:string)
                n273 = Index Array(array=w684) -> (element #1=w683:string, element #2=w678:string, element #3=w677:string, element #4=w676:string)  [unwired: 4 in]
                n274 = call <vilib>:"Trim Whitespace.vi"("string"=w680) -> ("trimmed string"=w681:string)  [unwired: 1 in]
                n275 = call "PADMINI_SHIFT_DATE.vi"("SHIFT"=w691) -> ("date/time string"=w673:string)  [unwired: 10 in]
                n276 = Format Into String(format string="Where BARCODE='%s' ", w681) -> (resulting string=w686:string)  [unwired: 2 in, 1 out]
                n277 = Bundle("date/time string"=w673, "Input 2"=w683, "Input 2"=w675, "Input 2"=w678, "Input 2"=w674, "Input 2"=w677, "Input 2"=w676, "Input 2"=w672, "Input 2"=w671) -> (w682:T22)  [unwired: 1 in]
                n278 = call <vilib>:"DB Tools Update Data.vi"("condition"=w686, "data"=w682, "error in (no error)"=w690, "columns"=string[] ["OP40_DATE", "OP40_RH_SCREW_Nm", "OP40_RH_STATUS", "OP40_LH_SCREW_Nm", "OP40_LH_STATUS", "OP40_DISPLACEMENT_mm", "OP40_STACK_LOAD_kg", "OP40_TOP_BEARING_CAMERA_STAUS", "OP40_FINAL_RESULT"], "table"=w688, "connection reference"=w689) -> ("error out"=w692:errorcluster, "connection reference out"=w693:T14)  [unwired: 4 in]
              }
              frame True {
                # "TRAC BYPASS"
                n279 = local read "SHIFT"() -> (w696:string)
                n280 = Index Array(array=w694) -> (element #2=w704:string, element #3=w703:string, element #4=w702:string, element #5=w701:string)  [unwired: 5 in, 1 out]
                n281 = call "PADMINI_SHIFT_DATE.vi"("SHIFT"=w696) -> ("date/time string"=w697:string)  [unwired: 10 in]
                n282 = Index Array(array=w695) -> (element #1=w698:string, element #2=w707:string, element #3=w706:string, element #4=w705:string)  [unwired: 4 in]
                n283 = Bundle("date/time string"=w697, "SHIFT"=w696, "Input 2"=w698, "Input 2"=w704, "Input 2"=w707, "Input 2"=w703, "Input 2"=w706, "Input 2"=w705, "Input 2"=w701, "Input 2"=w702) -> (w700:T23)  [unwired: 1 in]
                n284 = To Variant(anything=w700) -> (Variant=w699:variant)
                n285 = call <vilib>:"DB Tools Insert Data.vi"("data"=w699, "error in (no error)"=w712, "columns"=string[] ["DATE", "SHIFT", "ST4_SCREW1_DATA", "ST4_SCREW1_STATUS", "ST4_SCREW2_DATA", "ST4_SCREW2_STATUS", "ST4_DISPLACEMENT", "ST4_LOAD", "ST4_TOP_BEARING_CAMERA_STAUS", "ST4_FINAL_RST"], "table"="ST4_REPORT", "connection reference"=w713) -> ("error out"=w710:errorcluster, "connection reference out"=w711:T14)  [unwired: 5 in]
              }
            }
            n286 = call <vilib>:"Simple Error Handler.vi"("type of dialog (OK msg:1)"=w661, "error in (no error)"=w662) -> ("error out"=w660:errorcluster)  [unwired: 3 in, 4 out]
            n287 = call <vilib>:"Clear Errors.vi"("error in (no error)"=w660) -> ("error out"=w658:errorcluster)  [unwired: 5 in, 1 out]
            n288 = flat-sequence {
              tunnel: [w670] -> w648
              tunnel: w658 -> [w670]
              frame #0 {
                # "UPDATE op 20 save"
                n289 = global write "DATA LOG.vi" "OP 40 reset"(TRUE) -> ()
              }
            }
          }
          frame "SCAN5" {
            # "STATION OP 50"
            n290 = case shown="False" w720 {
              tunnel: w724 -> [w745 w751]
              tunnel: w723 -> [w738 w750]
              tunnel: w722 -> [w730 _]
              tunnel: [w740 w749] -> w719
              tunnel: [w739 w751] -> w721
              tunnel: [w731 "" ("trimmed string")] -> _
              frame False {
                n291 = call "PADMINI_AUTO_BARCODE_STRING 50.vi"("Enum"=enum16{"Read", "Write"}."Read", "error in (no error)"=w738) -> ("error out"=w737:errorcluster, "Input 2"=w733:string[])  [unwired: 8 in]
                n292 = Index Array(array=w733) -> (element=w732:string)  [unwired: 1 in]
                n293 = call <vilib>:"Trim Whitespace.vi"("string"=w732) -> ("trimmed string"=w731:string)  [unwired: 1 in]
                n294 = Format Into String(format string="WHERE BARCODE  ='%s'", w731) -> (resulting string=w734:string)  [unwired: 2 in, 1 out]
                n295 = call <vilib>:"DB Tools Select Data.vi"("condition"=w734, "error in (no error)"=w737, "columns"=string[] ["BARCODE", "OP40_FINAL_RESULT", "OP50_FINAL_RESULT"], "table"=w730, "connection reference"=w745) -> ("error out"=w743:errorcluster, "data"=w742:variant[][], "connection reference out"=w739:T14)  [unwired: 1 in]
                n296 = call "PADMINI_varient_to_data.vi"("error in (no error)"=w743, "data"=w742) -> ("error out"=w741:errorcluster, "Array"=w727:string[][])  [unwired: 8 in]
                n297 = Index Array(array=w727, index (row)=0 ("disabled index (col)")) -> (element=→"SCAN OP50":string[])  [unwired: 1 in]
                n298 = call "RESPONSE_LOGIC.vi"("Array"=w727) -> ("Not Found"=w726:i32[])  [unwired: 10 in]
                "OP50 STATUS" <- w726
                n299 = call "PADMINI_AUTO_BARCODE_STATUS 50.vi"("Enum"=enum16{"Read", "Write"}."Write", "error in (no error)"=w741, "I/P"=w726) -> ("error out"=w740:errorcluster)  [unwired: 7 in, 1 out]
              }
              frame True {
                w746 = i32[] [0, 0, 0, 0, 0]  # I/P
                n300 = call "PADMINI_AUTO_BARCODE_STATUS 50.vi"("Enum"=enum16{"Read", "Write"}."Write", "error in (no error)"=w750, "I/P"=w746) -> ("error out"=w749:errorcluster)  [unwired: 7 in, 1 out]
              }
            }
            n301 = flat-sequence {
              tunnel: [w753] -> w718
              tunnel: w719 -> [w753]
              frame #0 {
                # "UPDATE op 50 SCAN sTATUS"
                n302 = global write "DATA LOG.vi" "OP 50 Outputs"(TRUE) -> ()
              }
            }
          }
          frame "DATALOG5" {
            (unwired) string[] ["OP50_DATE", "OP50_NUT_TORQUE_Nm", "OP50_NUT_STATUS", "OP50_LH_MOTOR_SCREW_Nm", "OP50_LH_STATUS", "OP50_RH_MOTOR_SCREW_Nm", "OP50_RH_STATUS", "OP50_CAMERA_STATUS", "OP50_FINAL_RESULT"]
            w767 = T15 2 items=["no dialog", "OK message", "continue or stop message", "OK message + warnings", "continue/stop + warnings"] ("type of dialog (OK msg:1)")
            # "datalog of OP 50"
            n303 = call "PADMINI_AUTO_BARCODE_STRING 50.vi"("Enum"=enum16{"Read", "Write"}."Read", "error in (no error)"=w760) -> ("error out"=w762:errorcluster, "Input 2"=w756:string[])  [unwired: 8 in]
            n304 = call "PADMINI_AUTO_CYCLE VALUE 50.vi"("Enum"=enum16{"Read", "Write"}."Read", "error in (no error)"=w760) -> ("Input 2"=w758:sgl[])  [unwired: 8 in, 1 out]
            n305 = Number To Fractional String(number=w758, precision (6)=i16 2) -> (F-format string=w757:string[])  [unwired: 2 in]
            n306 = case shown="False" w772 {
              tunnel: w773 -> [w795 w817]
              tunnel: w762 -> [w796 w816]
              tunnel: [w799 w815] -> w770
              tunnel: [w798 w814] -> w768
              tunnel: w771 -> [w794 _]
              tunnel: w757 -> [w791 w801]
              tunnel: w756 -> [w787 w800]
              frame False {
                # "DO TRACEBILITY"
                n307 = Index Array(array=w787) -> (element #1=w788:string, element #2=w783:string, element #3=w781:string, element #4=w779:string, element #5=w778:string, element #6=w777:string)  [unwired: 6 in]
                n308 = local read "SHIFT"() -> (w797:string)
                n309 = Index Array(array=w791) -> (element #1=w784:string, element #2=w782:string, element #3=w780:string)  [unwired: 3 in]
                n310 = call <vilib>:"Trim Whitespace.vi"("string"=w788) -> ("trimmed string"=w789:string)  [unwired: 1 in]
                n311 = call "PADMINI_SHIFT_DATE.vi"("SHIFT"=w797) -> ("date/time string"=w786:string)  [unwired: 10 in]
                n312 = Format Into String(format string="Where BARCODE='%s' ", w789) -> (resulting string=w792:string)  [unwired: 2 in, 1 out]
                n313 = Bundle("date/time string"=w786, "Input 2"=w784, "Input 2"=w783, "Input 2"=w782, "Input 2"=w781, "Input 2"=w780, "Input 2"=w779, "Input 2"=w778, "Input 2"=w777) -> (w790:T22)  [unwired: 1 in]
                n314 = call <vilib>:"DB Tools Update Data.vi"("condition"=w792, "data"=w790, "error in (no error)"=w796, "columns"=string[] ["OP50_DATE", "OP50_NUT_TORQUE_Nm", "OP50_NUT_STATUS", "OP50_RH_MOTOR_SCREW_Nm", "OP50_RH_STATUS", "OP50_LH_MOTOR_SCREW_Nm", "OP50_LH_STATUS", "OP50_CAMERA_STATUS", "OP50_FINAL_RESULT"], "table"=w794, "connection reference"=w795) -> ("error out"=w798:errorcluster, "connection reference out"=w799:T14)  [unwired: 4 in]
              }
              frame True {
                # "TRAC BYPASS"
                n315 = local read "SHIFT"() -> (w802:string)
                n316 = Index Array(array=w800) -> (element #2=w806:string, element #3=w805:string, element #4=w810:string)  [unwired: 4 in, 1 out]
                n317 = Index Array(array=w801) -> (element #1=w809:string, element #2=w808:string, element #3=w807:string)  [unwired: 3 in]
                n318 = call "PADMINI_SHIFT_DATE.vi"("SHIFT"=w802) -> ("date/time string"=w803:string)  [unwired: 10 in]
                n319 = Bundle("date/time string"=w803, "SHIFT"=w802, "Input 2"=w809, "Input 2"=w806, "Input 2"=w808, "Input 2"=w805, "Input 2"=w807, "Input 2"=w810) -> (w804:T24)  [unwired: 1 in]
                n320 = To Variant(anything=w804) -> (Variant=w813:variant)
                n321 = call <vilib>:"DB Tools Insert Data.vi"("data"=w813, "error in (no error)"=w816, "columns"=string[] ["DATE", "SHIFT", "ST5_SCREW1_DATA", "ST5_SCREW1_STATUS", "ST5_SCREW2_DATA", "ST5_SCREW2_STATUS", "ST5_SCREW3_DATA", "ST5_FINAL_RST"], "table"="ST5_REPORT", "connection reference"=w817) -> ("error out"=w814:errorcluster, "connection reference out"=w815:T14)  [unwired: 5 in]
              }
            }
            n322 = call <vilib>:"Simple Error Handler.vi"("type of dialog (OK msg:1)"=w767, "error in (no error)"=w768) -> ("error out"=w766:errorcluster)  [unwired: 3 in, 4 out]
            n323 = call <vilib>:"Clear Errors.vi"("error in (no error)"=w766) -> ("error out"=w764:errorcluster)  [unwired: 5 in, 1 out]
            n324 = flat-sequence {
              tunnel: [w776] -> w755
              tunnel: w764 -> [w776]
              frame #0 {
                # "UPDATE op 20 save"
                n325 = global write "DATA LOG.vi" "OP 50 reset"(TRUE) -> ()
              }
            }
          }
          frame "SCAN6" {
            # "STATION OP 60"
            n326 = case shown="False" w824 {
              tunnel: w828 -> [w849 w855]
              tunnel: w827 -> [w842 w854]
              tunnel: w826 -> [_ _]
              tunnel: [w844 w853] -> w823
              tunnel: [w843 w855] -> w825
              tunnel: [w834 "" ("trimmed string")] -> _
              frame False {
                n327 = call "PADMINI_AUTO_BARCODE_STRING 60.vi"("Enum"=enum16{"Read", "Write"}."Read", "error in (no error)"=w842) -> ("error out"=w841:errorcluster, "Input 2"=w836:string[])  [unwired: 8 in]
                n328 = Index Array(array=w836) -> (element=w835:string)  [unwired: 1 in]
                n329 = call <vilib>:"Trim Whitespace.vi"("string"=w835) -> ("trimmed string"=w834:string)  [unwired: 1 in]
                n330 = Format Into String(format string="WHERE BARCODE  ='%s'", w834) -> (resulting string=w837:string)  [unwired: 2 in, 1 out]
                n331 = call <vilib>:"DB Tools Select Data.vi"("condition"=w837, "error in (no error)"=w841, "columns"=string[] ["BARCODE", "OP50_FINAL_RESULT", "OP60_FINAL_RESULT"], "table"="REPORT", "connection reference"=w849) -> ("error out"=w847:errorcluster, "data"=w846:variant[][], "connection reference out"=w843:T14)  [unwired: 1 in]
                n332 = call "PADMINI_varient_to_data.vi"("error in (no error)"=w847, "data"=w846) -> ("error out"=w845:errorcluster, "Array"=w831:string[][])  [unwired: 8 in]
                n333 = Index Array(array=w831, index (row)=0 ("disabled index (col)")) -> (element=→"SCAN OP60":string[])  [unwired: 1 in]
                n334 = call "RESPONSE_LOGIC.vi"("Array"=w831) -> ("Not Found"=w829:i32[])  [unwired: 10 in]
                "OP60 STATUS" <- w829
                n335 = call "PADMINI_AUTO_BARCODE_STATUS 60.vi"("Enum"=enum16{"Read", "Write"}."Write", "error in (no error)"=w845, "I/P"=w829) -> ("error out"=w844:errorcluster)  [unwired: 7 in, 1 out]
              }
              frame True {
                w850 = i32[] [0, 0, 0, 0, 0]  # I/P
                n336 = call "PADMINI_AUTO_BARCODE_STATUS 60.vi"("Enum"=enum16{"Read", "Write"}."Write", "error in (no error)"=w854, "I/P"=w850) -> ("error out"=w853:errorcluster)  [unwired: 7 in, 1 out]
              }
            }
            n337 = flat-sequence {
              tunnel: [w857] -> w822
              tunnel: w823 -> [w857]
              frame #0 {
                # "UPDATE op 60 SCAN sTATUS"
                n338 = global write "DATA LOG.vi" "OP 60 Outputs"(TRUE) -> ()
              }
            }
          }
          frame "DATALOG6" {
            w871 = T15 2 items=["no dialog", "OK message", "continue or stop message", "OK message + warnings", "continue/stop + warnings"] ("type of dialog (OK msg:1)")
            # "datalog of OP 60"
            n339 = call "PADMINI_AUTO_BARCODE_STRING 60.vi"("Enum"=enum16{"Read", "Write"}."Read", "error in (no error)"=w863) -> ("error out"=w865:errorcluster, "Input 2"=w859:string[])  [unwired: 8 in]
            n340 = call "PADMINI_AUTO_CYCLE VALUE 60.vi"("Enum"=enum16{"Read", "Write"}."Read", "error in (no error)"=w863) -> ("Input 2"=w861:sgl[])  [unwired: 8 in, 1 out]
            n341 = Number To Fractional String(number=w861, precision (6)=i16 2) -> (F-format string=w860:string[])  [unwired: 2 in]
            n342 = case shown="False" w876 {
              tunnel: w877 -> [w904 w932]
              tunnel: w865 -> [w905 w931]
              tunnel: [w908 w930] -> w874
              tunnel: [w907 w929] -> w872
              tunnel: w875 -> [w903 _]
              tunnel: w860 -> [w899 w912]
              tunnel: w859 -> [w895 w911]
              frame False {
                # "DO TRACEBILITY"
                n343 = Index Array(array=w895) -> (element #1=w896:string, element #2=w887:string, element #3=w886:string, element #4=w885:string, element #5=w884:string, element #6=w883:string, element #7=w882:string, element #8=w881:string)  [unwired: 8 in]
                n344 = local read "SHIFT"() -> (w906:string)
                n345 = Index Array(array=w899) -> (element #1=w893:string, element #2=w892:string, element #3=w891:string, element #4=w890:string, element #5=w889:string, element #6=w888:string)  [unwired: 6 in]
                n346 = call <vilib>:"Trim Whitespace.vi"("string"=w896) -> ("trimmed string"=w897:string)  [unwired: 1 in]
                n347 = call "PADMINI_SHIFT_DATE.vi"("SHIFT"=w906) -> ("date/time string"=w894:string)  [unwired: 10 in]
                n348 = Format Into String(format string="Where BARCODE='%s' ", w897) -> (resulting string=w901:string)  [unwired: 2 in, 1 out]
                n349 = Bundle("date/time string"=w894, "Input 2"=w893, "Input 2"=w887, "Input 2"=w892, "Input 2"=w886, "Input 2"=w891, "Input 2"=w885, "Input 2"=w890, "Input 2"=w884, "Input 2"=w889, "Input 2"=w883, "Input 2"=w888, "Input 2"=w882, "Input 2"=w881) -> (w898:T25)  [unwired: 1 in]
                n350 = call <vilib>:"DB Tools Update Data.vi"("condition"=w901, "data"=w898, "error in (no error)"=w905, "columns"=string[] ["OP60_DATE", "OP60_SCREW1_DATA_Nm", "OP60_SCREW1_STATUS", "OP60_SCREW2_DATA_Nm", "OP60_SCREW2_STATUS", "OP60_SCREW3_DATA_Nm", "OP60_SCREW3_STATUS", "OP60_SCREW4_DATA_Nm", "OP60_SCREW4_STATUS", "OP60_SCREW5_DATA_Nm", "OP60_SCREW5_STATUS", "OP60_SCREW6_DATA_Nm", "OP60_SCREW6_STATUS", "OP60_FINAL_RESULT"], "table"=w903, "connection reference"=w904) -> ("error out"=w907:errorcluster, "connection reference out"=w908:T14)  [unwired: 4 in]
              }
              frame True {
                # "TRAC BYPASS"
                n351 = local read "SHIFT"() -> (w909:string)
                n352 = call "PADMINI_SHIFT_DATE.vi"("SHIFT"=w909) -> ("date/time string"=w910:string)  [unwired: 10 in]
                n353 = Index Array(array=w911) -> (element #2=w920:string, element #3=w919:string, element #4=w918:string, element #5=w916:string, element #6=w924:string, element #7=w925:string)  [unwired: 7 in, 1 out]
                n354 = Index Array(array=w912) -> (element #1=w923:string, element #2=w922:string, element #3=w921:string, element #4=w917:string, element #5=w915:string, element #6=w914:string)  [unwired: 6 in]
                n355 = Bundle("date/time string"=w910, "SHIFT"=w909, "Input 2"=w923, "Input 2"=w920, "Input 2"=w922, "Input 2"=w919, "Input 2"=w921, "Input 2"=w918, "Input 2"=w917, "Input 2"=w916, "Input 2"=w915, "Input 2"=w914, "Input 2"=w924, "Input 2"=w925) -> (w913:T26)  [unwired: 1 in]
                n356 = To Variant(anything=w913) -> (Variant=w928:variant)
                n357 = call <vilib>:"DB Tools Insert Data.vi"("data"=w928, "error in (no error)"=w931, "columns"=string[] ["DATE", "SHIFT", "ST6_SCREW1_DATA", "ST6_SCREW1_STATUS", "ST6_SCREW2_DATA", "ST6_SCREW2_STATUS", "ST6_SCREW3_DATA", "ST6_SCREW3_STATUS", "ST6_SCREW4_DATA", "ST6_SCREW4_STATUS", "ST6_SCREW5_DATA", "ST6_SCREW5_STATUS", "ST6_SCREW6_DATA", "ST6_SCREW6_STATUS", "ST6_FINAL_RST"], "table"="ST6_REPORT", "connection reference"=w932) -> ("error out"=w929:errorcluster, "connection reference out"=w930:T14)  [unwired: 5 in]
              }
            }
            n358 = call <vilib>:"Simple Error Handler.vi"("type of dialog (OK msg:1)"=w871, "error in (no error)"=w872) -> ("error out"=w870:errorcluster)  [unwired: 3 in, 4 out]
            n359 = call <vilib>:"Clear Errors.vi"("error in (no error)"=w870) -> ("error out"=w868:errorcluster)  [unwired: 5 in, 1 out]
            n360 = flat-sequence {
              tunnel: [w880] -> w858
              tunnel: w868 -> [w880]
              frame #0 {
                # "UPDATE op 20 save"
                n361 = global write "DATA LOG.vi" "OP 60 reset"(TRUE) -> ()
              }
            }
          }
          frame "SCAN7" {
            # "STATION OP 70"
            n362 = case shown="False" w939 {
              tunnel: w943 -> [w964 w970]
              tunnel: w942 -> [w957 w969]
              tunnel: w941 -> [w949 _]
              tunnel: [w959 w968] -> w938
              tunnel: [w958 w970] -> w940
              tunnel: [w950 "" ("trimmed string")] -> _
              frame False {
                n363 = call "PADMINI_AUTO_BARCODE_STRING 70.vi"("Enum"=enum16{"Read", "Write"}."Read", "error in (no error)"=w957) -> ("error out"=w956:errorcluster, "Input 2"=w952:string[])  [unwired: 8 in]
                n364 = Index Array(array=w952) -> (element=w951:string)  [unwired: 1 in]
                n365 = call <vilib>:"Trim Whitespace.vi"("string"=w951) -> ("trimmed string"=w950:string)  [unwired: 1 in]
                n366 = Format Into String(format string="WHERE BARCODE  ='%s'", w950) -> (resulting string=w953:string)  [unwired: 2 in, 1 out]
                n367 = call <vilib>:"DB Tools Select Data.vi"("condition"=w953, "error in (no error)"=w956, "columns"=string[] ["BARCODE", "OP60_FINAL_RESULT", "OP70_FINAL_RESULT"], "table"=w949, "connection reference"=w964) -> ("error out"=w962:errorcluster, "data"=w961:variant[][], "connection reference out"=w958:T14)  [unwired: 1 in]
                n368 = call "PADMINI_varient_to_data.vi"("error in (no error)"=w962, "data"=w961) -> ("error out"=w960:errorcluster, "Array"=w946:string[][])  [unwired: 8 in]
                n369 = Index Array(array=w946, index (row)=0 ("disabled index (col)")) -> (element=→"SCAN OP70":string[])  [unwired: 1 in]
                n370 = call "RESPONSE_LOGIC.vi"("Array"=w946) -> ("Not Found"=w944:i32[])  [unwired: 10 in]
                "OP70 STATUS" <- w944
                n371 = call "PADMINI_AUTO_BARCODE_STATUS 70.vi"("Enum"=enum16{"Read", "Write"}."Write", "error in (no error)"=w960, "I/P"=w944) -> ("error out"=w959:errorcluster)  [unwired: 7 in, 1 out]
              }
              frame True {
                w965 = i32[] [0, 0, 0, 0, 0]  # I/P
                n372 = call "PADMINI_AUTO_BARCODE_STATUS 70.vi"("Enum"=enum16{"Read", "Write"}."Write", "error in (no error)"=w969, "I/P"=w965) -> ("error out"=w968:errorcluster)  [unwired: 7 in, 1 out]
              }
            }
            n373 = flat-sequence {
              tunnel: [w972] -> w937
              tunnel: w938 -> [w972]
              frame #0 {
                # "UPDATE op 70 SCAN sTATUS"
                n374 = global write "DATA LOG.vi" "OP 70 Outputs"(TRUE) -> ()
              }
            }
          }
          frame "DATALOG7" {
            # "datalog of OP 70"
            n375 = call "PADMINI_AUTO_BARCODE_STRING 70.vi"("Enum"=enum16{"Read", "Write"}."Read", "error in (no error)"=w978) -> ("error out"=w980:errorcluster, "Input 2"=w974:string[])  [unwired: 8 in]
            n376 = call "PADMINI_AUTO_CYCLE VALUE 70.vi"("Enum"=enum16{"Read", "Write"}."Read", "error in (no error)"=w978) -> ("Input 2"=w976:sgl[])  [unwired: 8 in, 1 out]
            n377 = Number To Fractional String(number=w976, precision (6)=i16 4) -> (F-format string=w975:string[])  [unwired: 2 in]
            n378 = case shown="False" w988 {
              tunnel: w989 -> [w1007 w1025]
              tunnel: w980 -> [w1008 w1024]
              tunnel: [w1010 w1023] -> w986
              tunnel: [w1009 w1022] -> w984
              tunnel: w987 -> [w1006 _]
              tunnel: w975 -> [w1002 w1012]
              tunnel: w974 -> [w997 w1011]
              frame False {
                # "DO TRACEBILITY"
                n379 = Index Array(array=w997) -> (element #1=w998:string, element #2=w996:string)  [unwired: 2 in]
                n380 = call <vilib>:"Trim Whitespace.vi"("string"=w998) -> ("trimmed string"=w999:string)  [unwired: 1 in]
                n381 = local read "SHIFT"() -> (w994:string)
                n382 = Index Array(array=w1002) -> (element #1=w1001:string, element #2=w995:string)  [unwired: 2 in]
                n383 = call "PADMINI_SHIFT_DATE.vi"("SHIFT"=w994) -> ("date/time string"=w993:string)  [unwired: 10 in]
                n384 = Bundle("date/time string"=w993, "Input 2"=w1001, "Input 2"=w995, "Input 2"=w996) -> (w1000:T27)  [unwired: 1 in]
                n385 = Format Into String(format string="Where BARCODE='%s' ", w999) -> (resulting string=w1004:string)  [unwired: 2 in, 1 out]
                n386 = call <vilib>:"DB Tools Update Data.vi"("condition"=w1004, "data"=w1000, "error in (no error)"=w1008, "columns"=string[] ["OP70_DATE", "OP70_FULL_OPEN", "OP70_FULL_CLOSE", "OP70_FINAL_RESULT"], "table"=w1006, "connection reference"=w1007) -> ("error out"=w1009:errorcluster, "connection reference out"=w1010:T14)  [unwired: 4 in]
              }
              frame True {
                # "TRAC BYPASS"
                n387 = local read "SHIFT"() -> (w1013:string)
                n388 = call "PADMINI_SHIFT_DATE.vi"("SHIFT"=w1013) -> ("date/time string"=w1014:string)  [unwired: 10 in]
                n389 = Index Array(array=w1011) -> (element #2=w1017:string)  [unwired: 2 in, 1 out]
                n390 = Index Array(array=w1012) -> (element #1=w1018:string, element #2=w1016:string)  [unwired: 2 in]
                n391 = Bundle("date/time string"=w1014, "SHIFT"=w1013, "Input 2"=w1018, "Input 2"=w1016, "Input 2"=w1017) -> (w1015:T28)  [unwired: 1 in]
                n392 = To Variant(anything=w1015) -> (Variant=w1021:variant)
                n393 = call <vilib>:"DB Tools Insert Data.vi"("data"=w1021, "error in (no error)"=w1024, "columns"=string[] ["DATE_OP70", "SHIFT", "OP70_FULL_OPEN", "OP70_FULL_CLOSE", "OP70_FINAL_RST"], "table"="ST7_REPORT", "connection reference"=w1025) -> ("error out"=w1022:errorcluster, "connection reference out"=w1023:T14)  [unwired: 5 in]
              }
            }
            n394 = flat-sequence {
              tunnel: [w992] -> w973
              tunnel: w984 -> [w992]
              frame #0 {
                # "UPDATE op 20 save"
                n395 = global write "DATA LOG.vi" "OP 70 reset"(TRUE) -> ()
              }
            }
          }
          frame "SCAN8" {
            # "STATION OP 80"
            n396 = case shown="False" w1032 {
              tunnel: w1036 -> [w1057 w1063]
              tunnel: w1035 -> [w1050 w1062]
              tunnel: w1034 -> [w1042 _]
              tunnel: [w1052 w1061] -> w1031
              tunnel: [w1051 w1063] -> w1033
              tunnel: [w1043 "" ("trimmed string")] -> _
              frame False {
                (unwired) "REPORT"
                n397 = call "PADMINI_AUTO_BARCODE_STRING 80.vi"("Enum"=enum16{"Read", "Write"}."Read", "error in (no error)"=w1050) -> ("error out"=w1049:errorcluster, "Input 2"=w1045:string[])  [unwired: 8 in]
                n398 = Index Array(array=w1045) -> (element=w1044:string)  [unwired: 1 in]
                n399 = call <vilib>:"Trim Whitespace.vi"("string"=w1044) -> ("trimmed string"=w1043:string)  [unwired: 1 in]
                n400 = Format Into String(format string="WHERE BARCODE  ='%s'", w1043) -> (resulting string=w1046:string)  [unwired: 2 in, 1 out]
                n401 = call <vilib>:"DB Tools Select Data.vi"("condition"=w1046, "error in (no error)"=w1049, "columns"=string[] ["BARCODE", "OP70_FINAL_RESULT", "OP80_FINAL_RESULT"], "table"=w1042, "connection reference"=w1057) -> ("error out"=w1055:errorcluster, "data"=w1054:variant[][], "connection reference out"=w1051:T14)  [unwired: 1 in]
                n402 = call "PADMINI_varient_to_data.vi"("error in (no error)"=w1055, "data"=w1054) -> ("error out"=w1053:errorcluster, "Array"=w1039:string[][])  [unwired: 8 in]
                n403 = Index Array(array=w1039, index (row)=0 ("disabled index (col)")) -> (element=→"SCAN OP80":string[])  [unwired: 1 in]
                n404 = call "RESPONSE_LOGIC.vi"("Array"=w1039) -> ("Not Found"=w1038:i32[])  [unwired: 10 in]
                "OP80 STATUS" <- w1038
                n405 = call "PADMINI_AUTO_BARCODE_STATUS 80.vi"("Enum"=enum16{"Read", "Write"}."Write", "error in (no error)"=w1053, "I/P"=w1038) -> ("error out"=w1052:errorcluster)  [unwired: 7 in, 1 out]
              }
              frame True {
                w1058 = i32[] [0, 0, 0, 0, 0]  # I/P
                n406 = call "PADMINI_AUTO_BARCODE_STATUS 80.vi"("Enum"=enum16{"Read", "Write"}."Write", "error in (no error)"=w1062, "I/P"=w1058) -> ("error out"=w1061:errorcluster)  [unwired: 7 in, 1 out]
              }
            }
            n407 = flat-sequence {
              tunnel: [w1065] -> w1030
              tunnel: w1031 -> [w1065]
              frame #0 {
                # "UPDATE op 80 SCAN sTATUS"
                n408 = global write "DATA LOG.vi" "OP 80 Outputs"(TRUE) -> ()
              }
            }
          }
          frame "DATALOG8" {
            w1080 = T15 2 items=["no dialog", "OK message", "continue or stop message", "OK message + warnings", "continue/stop + warnings"] ("type of dialog (OK msg:1)")
            # "datalog of OP 80"
            n409 = call "PADMINI_AUTO_BARCODE_STRING 80.vi"("Enum"=enum16{"Read", "Write"}."Read", "error in (no error)"=w1072) -> ("error out"=w1074:errorcluster, "Input 2"=w1068:string[])  [unwired: 8 in]
            n410 = call "PADMINI_AUTO_CYCLE VALUE 80.vi"("Enum"=enum16{"Read", "Write"}."Read", "error in (no error)"=w1072) -> ("Input 2"=w1070:sgl[])  [unwired: 8 in, 1 out]
            n411 = Number To Fractional String(number=w1070, precision (6)=i16 2) -> (F-format string=w1069:string[])  [unwired: 2 in]
            n412 = case shown="True" w1066 {
              tunnel: w1085 -> [w1103 w1122]
              tunnel: w1074 -> [w1104 w1121]
              tunnel: [w1106 w1120] -> w1083
              tunnel: [w1105 w1119] -> w1081
              tunnel: w1084 -> [w1102 w1107]
              tunnel: w1069 -> [w1098 w1112]
              tunnel: w1068 -> [w1094 w1113]
              frame False {
                # "DO TRACEBILITY"
                n413 = Index Array(array=w1094) -> (element #1=w1095:string, element #2=w1090:string, element #3=w1089:string)  [unwired: 3 in]
                n414 = call <vilib>:"Trim Whitespace.vi"("string"=w1095) -> ("trimmed string"=w1096:string)  [unwired: 1 in]
                n415 = local read "SHIFT"() -> (w1093:string)
                n416 = Index Array(array=w1098) -> (element=w1091:string)  [unwired: 1 in]
                n417 = call "PADMINI_SHIFT_DATE.vi"("SHIFT"=w1093) -> ("date/time string"=w1092:string)  [unwired: 10 in]
                n418 = Bundle("date/time string"=w1092, "Input 2"=w1090, "Input 2"=w1091, "Input 2"=w1089) -> (w1097:T27)  [unwired: 1 in]
                n419 = Format Into String(format string="Where BARCODE='%s' ", w1096) -> (resulting string=w1100:string)  [unwired: 2 in, 1 out]
                n420 = call <vilib>:"DB Tools Update Data.vi"("condition"=w1100, "data"=w1097, "error in (no error)"=w1104, "columns"=string[] ["OP80_DATE", "OP80_LOCTITE_STATUS", "OP80_PLUG_PRESS_LOAD_kg", "OP80_FINAL_RESULT"], "table"=w1102, "connection reference"=w1103) -> ("error out"=w1105:errorcluster, "connection reference out"=w1106:T14)  [unwired: 4 in]
              }
              frame True {
                (unwired) "ST8_REPORT"
                # "TRAC BYPASS"
                n421 = local read "SHIFT"() -> (w1109:string)
                n422 = call "PADMINI_SHIFT_DATE.vi"("SHIFT"=w1109) -> ("date/time string"=w1108:string)  [unwired: 10 in]
                n423 = Index Array(array=w1113) -> (element #1=w1110:string, element #2=w1117:string, element #3=w1116:string)  [unwired: 3 in]
                n424 = Index Array(array=w1112) -> (element=w1115:string)  [unwired: 1 in]
                n425 = Bundle("Input 2"=w1110, "SHIFT"=w1109, "date/time string"=w1108, "Input 2"=w1115, "Input 2"=w1117, "Input 2"=w1116) -> (w1114:T29)  [unwired: 1 in]
                n426 = To Variant(anything=w1114) -> (Variant=w1118:variant)
                n427 = call <vilib>:"DB Tools Insert Data.vi"("data"=w1118, "error in (no error)"=w1121, "columns"=string[] ["BARCODE", "SHIFT", "OP80_DATE", "OP80_LOCTITE_STATUS", "OP80_PLUG_PRESS_LOAD_kg", "OP80_FINAL_RESULT"], "table"=w1107, "connection reference"=w1122) -> ("error out"=w1119:errorcluster, "connection reference out"=w1120:T14)  [unwired: 5 in]
              }
            }
            n428 = call <vilib>:"Simple Error Handler.vi"("type of dialog (OK msg:1)"=w1080, "error in (no error)"=w1081) -> ("error out"=w1079:errorcluster)  [unwired: 3 in, 4 out]
            n429 = call <vilib>:"Clear Errors.vi"("error in (no error)"=w1079) -> ("error out"=w1077:errorcluster)  [unwired: 5 in, 1 out]
            n430 = flat-sequence {
              tunnel: [w1088] -> w1067
              tunnel: w1077 -> [w1088]
              frame #0 {
                # "UPDATE op 20 save"
                n431 = global write "DATA LOG.vi" "OP 80 reset"(TRUE) -> ()
              }
            }
          }
          frame "SCAN9" {
            # "STATION OP 90"
            n432 = case shown="False" w1129 {
              tunnel: w1133 -> [w1154 w1160]
              tunnel: w1132 -> [w1147 w1159]
              tunnel: w1131 -> [w1139 _]
              tunnel: [w1149 w1158] -> w1128
              tunnel: [w1148 w1160] -> w1130
              tunnel: [w1140 "" ("trimmed string")] -> _
              frame False {
                (unwired) "REPORT"
                n433 = call "PADMINI_AUTO_BARCODE_STRING 90.vi"("Enum"=enum16{"Read", "Write"}."Read", "error in (no error)"=w1147) -> ("error out"=w1146:errorcluster, "Input 2"=w1142:string[])  [unwired: 8 in]
                n434 = Index Array(array=w1142) -> (element=w1141:string)  [unwired: 1 in]
                n435 = call <vilib>:"Trim Whitespace.vi"("string"=w1141) -> ("trimmed string"=w1140:string)  [unwired: 1 in]
                n436 = Format Into String(format string="WHERE BARCODE  ='%s'", w1140) -> (resulting string=w1143:string)  [unwired: 2 in, 1 out]
                n437 = call <vilib>:"DB Tools Select Data.vi"("condition"=w1143, "error in (no error)"=w1146, "columns"=string[] ["BARCODE", "OP80_FINAL_RESULT", "OP90_FINAL_RESULT"], "table"=w1139, "connection reference"=w1154) -> ("error out"=w1152:errorcluster, "data"=w1151:variant[][], "connection reference out"=w1148:T14)  [unwired: 1 in]
                n438 = call "PADMINI_varient_to_data.vi"("error in (no error)"=w1152, "data"=w1151) -> ("error out"=w1150:errorcluster, "Array"=w1136:string[][])  [unwired: 8 in]
                n439 = Index Array(array=w1136, index (row)=0 ("disabled index (col)")) -> (element=→"SCAN OP90":string[])  [unwired: 1 in]
                n440 = call "RESPONSE_LOGIC.vi"("Array"=w1136) -> ("Not Found"=w1134:i32[])  [unwired: 10 in]
                "OP90 STATUS" <- w1134
                n441 = call "PADMINI_AUTO_BARCODE_STATUS 90.vi"("Enum"=enum16{"Read", "Write"}."Write", "error in (no error)"=w1150, "I/P"=w1134) -> ("error out"=w1149:errorcluster)  [unwired: 7 in, 1 out]
              }
              frame True {
                w1155 = i32[] [0, 0, 0, 0, 0]  # I/P
                n442 = call "PADMINI_AUTO_BARCODE_STATUS 90.vi"("Enum"=enum16{"Read", "Write"}."Write", "error in (no error)"=w1159, "I/P"=w1155) -> ("error out"=w1158:errorcluster)  [unwired: 7 in, 1 out]
              }
            }
            n443 = flat-sequence {
              tunnel: [w1162] -> w1127
              tunnel: w1128 -> [w1162]
              frame #0 {
                # "UPDATE op 90 SCAN sTATUS"
                n444 = global write "DATA LOG.vi" "OP 90 Outputs"(TRUE) -> ()
              }
            }
          }
          frame "DATALOG9" {
            w1176 = T15 2 items=["no dialog", "OK message", "continue or stop message", "OK message + warnings", "continue/stop + warnings"] ("type of dialog (OK msg:1)")
            # "datalog of OP 90"
            n445 = call "PADMINI_AUTO_BARCODE_STRING 90.vi"("Enum"=enum16{"Read", "Write"}."Read", "error in (no error)"=w1168) -> ("error out"=w1170:errorcluster, "Input 2"=w1165:string[])  [unwired: 8 in]
            n446 = call "PADMINI_AUTO_CYCLE VALUE 90.vi"("Enum"=enum16{"Read", "Write"}."Read", "error in (no error)"=w1168) -> ("Input 2"=w1164:sgl[])  [unwired: 8 in, 1 out]
            n447 = Number To Fractional String(number=w1164, precision (6)=i16 2) -> (F-format string=w1166:string[])  [unwired: 2 in]
            n448 = case shown="False" w1181 {
              tunnel: w1182 -> [w1201 w1220]
              tunnel: w1170 -> [w1202 w1219]
              tunnel: [w1204 w1218] -> w1179
              tunnel: [w1203 w1217] -> w1177
              tunnel: w1180 -> [w1200 _]
              tunnel: w1166 -> [w1196 w1209]
              tunnel: w1165 -> [w1192 w1208]
              frame False {
                # "DO TRACEBILITY"
                n449 = Index Array(array=w1192) -> (element #1=w1193:string, element #2=w1190:string, element #3=w1188:string)  [unwired: 3 in]
                n450 = call <vilib>:"Trim Whitespace.vi"("string"=w1193) -> ("trimmed string"=w1194:string)  [unwired: 1 in]
                n451 = local read "SHIFT"() -> (w1187:string)
                n452 = Index Array(array=w1196) -> (element #1=w1191:string, element #2=w1189:string)  [unwired: 2 in]
                n453 = call "PADMINI_SHIFT_DATE.vi"("SHIFT"=w1187) -> ("date/time string"=w1186:string)  [unwired: 10 in]
                n454 = Bundle("date/time string"=w1186, "Input 2"=w1191, "Input 2"=w1190, "Input 2"=w1189, "Input 2"=w1188) -> (w1195:T20)  [unwired: 1 in]
                n455 = Format Into String(format string="Where BARCODE='%s' ", w1194) -> (resulting string=w1198:string)  [unwired: 2 in, 1 out]
                n456 = call <vilib>:"DB Tools Update Data.vi"("condition"=w1198, "data"=w1195, "error in (no error)"=w1202, "columns"=string[] ["OP90_DATE", "OP90_SEAT_LEAK_LP", "OP90_SEAT_STATUS", "OP90_STEAM_LEAK_sccm", "OP90_FINAL_RESULT"], "table"=w1200, "connection reference"=w1201) -> ("error out"=w1203:errorcluster, "connection reference out"=w1204:T14)  [unwired: 4 in]
              }
              frame True {
                # "TRAC BYPASS"
                n457 = local read "SHIFT"() -> (w1205:string)
                n458 = call "PADMINI_SHIFT_DATE.vi"("SHIFT"=w1205) -> ("date/time string"=w1206:string)  [unwired: 10 in]
                n459 = Index Array(array=w1208) -> (element #2=w1213:string, element #3=w1211:string)  [unwired: 3 in, 1 out]
                n460 = Index Array(array=w1209) -> (element #1=w1214:string, element #2=w1212:string)  [unwired: 2 in]
                n461 = Bundle("date/time string"=w1206, "SHIFT"=w1205, "Input 2"=w1214, "Input 2"=w1213, "Input 2"=w1212, "Input 2"=w1211) -> (w1210:T21)  [unwired: 1 in]
                n462 = To Variant(anything=w1210) -> (Variant=w1216:variant)
                n463 = call <vilib>:"DB Tools Insert Data.vi"("data"=w1216, "error in (no error)"=w1219, "columns"=string[] ["DATE", "SHIFT", "ST9_SEAT_LT_DATA", "ST9_SEAT_STATUS", "ST9_STEAM_LT_DATA", "ST9_FINAL_RST"], "table"="ST9_REPORT", "connection reference"=w1220) -> ("error out"=w1217:errorcluster, "connection reference out"=w1218:T14)  [unwired: 5 in]
              }
            }
            n464 = call <vilib>:"Simple Error Handler.vi"("type of dialog (OK msg:1)"=w1176, "error in (no error)"=w1177) -> ("error out"=w1175:errorcluster)  [unwired: 3 in, 4 out]
            n465 = call <vilib>:"Clear Errors.vi"("error in (no error)"=w1175) -> ("error out"=w1173:errorcluster)  [unwired: 5 in, 1 out]
            n466 = flat-sequence {
              tunnel: [w1185] -> w1163
              tunnel: w1173 -> [w1185]
              frame #0 {
                # "UPDATE op 20 save"
                n467 = global write "DATA LOG.vi" "OP 90 reset"(TRUE) -> ()
              }
            }
          }
          frame "SCAN10" {
            # "STATION OP 10"
            n468 = case shown="False" w1227 {
              tunnel: w1231 -> [w1252 w1258]
              tunnel: w1230 -> [w1246 w1257]
              tunnel: w1229 -> [w1238 _]
              tunnel: [w1236 w1256] -> w1226
              tunnel: [w1247 w1258] -> w1228
              tunnel: [w1239 "" ("trimmed string")] -> _
              frame False {
                (unwired) "REPORT"
                n469 = call "PADMINI_AUTO_BARCODE_STRING 100.vi"("Enum"=enum16{"Read", "Write"}."Read", "error in (no error)"=w1246) -> ("error out"=w1245:errorcluster, "Input 2"=w1241:string[])  [unwired: 8 in]
                n470 = Index Array(array=w1241) -> (element=w1240:string)  [unwired: 1 in]
                n471 = call <vilib>:"Trim Whitespace.vi"("string"=w1240) -> ("trimmed string"=w1239:string)  [unwired: 1 in]
                n472 = Format Into String(format string="WHERE BARCODE  ='%s'", w1239) -> (resulting string=w1242:string)  [unwired: 2 in, 1 out]
                n473 = call <vilib>:"DB Tools Select Data.vi"("condition"=w1242, "error in (no error)"=w1245, "columns"=string[] ["BARCODE", "OP90_FINAL_RESULT", "OP100_FINAL_RESULT"], "table"=w1238, "connection reference"=w1252) -> ("error out"=w1250:errorcluster, "data"=w1249:variant[][], "connection reference out"=w1247:T14)  [unwired: 1 in]
                n474 = call "PADMINI_varient_to_data.vi"("error in (no error)"=w1250, "data"=w1249) -> ("error out"=w1248:errorcluster, "Array"=w1234:string[][])  [unwired: 8 in]
                n475 = Index Array(array=w1234, index (row)=0 ("disabled index (col)")) -> (element=→"SCAN OP100":string[])  [unwired: 1 in]
                n476 = call "RESPONSE_LOGIC.vi"("Array"=w1234) -> ("Not Found"=w1232:i32[])  [unwired: 10 in]
                "OP100 STATUS" <- w1232
                n477 = call "PADMINI_AUTO_BARCODE_STATUS 100.vi"("Enum"=enum16{"Read", "Write"}."Write", "error in (no error)"=w1248, "I/P"=w1232) -> ("error out"=w1236:errorcluster)  [unwired: 7 in, 1 out]
              }
              frame True {
                w1253 = i32[] [0, 0, 0, 0, 0]  # I/P
                n478 = call "PADMINI_AUTO_BARCODE_STATUS 100.vi"("Enum"=enum16{"Read", "Write"}."Write", "error in (no error)"=w1257, "I/P"=w1253) -> ("error out"=w1256:errorcluster)  [unwired: 7 in, 1 out]
              }
            }
            n479 = flat-sequence {
              tunnel: [w1260] -> w1225
              tunnel: w1226 -> [w1260]
              frame #0 {
                # "UPDATE op 100 SCAN sTATUS"
                n480 = global write "DATA LOG.vi" "OP 100 Outputs"(TRUE) -> ()
              }
            }
          }
          frame "SCAN11" {
            # "STATION OP 110"
            n481 = case shown="False" w1267 {
              tunnel: w1271 -> [w1298 w1308]
              tunnel: w1270 -> [w1291 w1307]
              tunnel: w1269 -> [w1283 _]
              tunnel: [w1293 w1306] -> w1266
              tunnel: [w1292 w1308] -> w1268
              frame False {
                (unwired) "REPORT"
                # "OP100 OK\nOP 100 NG"
                n482 = call "PADMINI_AUTO_BARCODE_STRING 100.vi"("Enum"=enum16{"Read", "Write"}."Read", "error in (no error)"=w1291) -> ("error out"=w1290:errorcluster, "Input 2"=w1285:string[])  [unwired: 8 in]
                n483 = Index Array(array=w1285) -> (element=w1284:string)  [unwired: 1 in]
                n484 = call <vilib>:"Trim Whitespace.vi"("string"=w1284) -> ("trimmed string"=w1286:string)  [unwired: 1 in]
                n485 = Format Into String(format string="WHERE BARCODE  ='%s'", w1286) -> (resulting string=w1287:string)  [unwired: 2 in, 1 out]
                n486 = call <vilib>:"DB Tools Select Data.vi"("condition"=w1287, "error in (no error)"=w1290, "columns"=string[] ["BARCODE", "OP100_FINAL_RESULT"], "table"=w1283, "connection reference"=w1298) -> ("error out"=w1296:errorcluster, "data"=w1295:variant[][], "connection reference out"=w1292:T14)  [unwired: 1 in]
                n487 = call "PADMINI_varient_to_data.vi"("error in (no error)"=w1296, "data"=w1295) -> ("error out"=w1294:errorcluster, "Array"=w1274:string[][])  [unwired: 8 in]
                n488 = Index Array(array=w1274, index (row)=0 ("disabled index (col)")) -> (element=w1273:string[])  [unwired: 1 in]
                "SCAN OP110" <- w1273
                n489 = Index Array(array=w1273) -> (element #1=w1281:string, element #2=w1278:string)  [unwired: 2 in]
                n490 = Equal?(x="", y=w1281) -> (x = y?=w1280:bool)
                n491 = Equal?(x=w1278, y="OK") -> (x = y?=w1279:bool)
                n492 = case shown="True" w1280 {
                  tunnel: w1279 -> [w1299 _]
                  tunnel: [w1300 w1303] -> w1272
                  frame False {
                    # "BARCODE FOUND"
                    n493 = case shown="False" w1299 {
                      tunnel: [w1301 w1302] -> w1300
                      frame False {
                        w1301 = i32[] [0, 1]  # OK
                        # "CT ST REPEAT NG & EMPTY"
                      }
                      frame True {
                        w1302 = i32[] [1, 0]  # NG
                        # "CT ST REPEAT EMPTY"
                      }
                    }
                  }
                  frame True {
                    w1303 = i32[] [0, 1]  # Not Found
                    # "nO BARCODE FOUND"
                  }
                }
                "OP110 STATUS" <- w1272
                n494 = call "PADMINI_AUTO_BARCODE_STATUS 110.vi"("Enum"=enum16{"Read", "Write"}."Write", "error in (no error)"=w1294, "I/P"=w1272) -> ("error out"=w1293:errorcluster)  [unwired: 7 in, 1 out]
              }
              frame True {
                w1304 = i32[] [0, 0, 0, 0, 0]  # I/P
                n495 = call "PADMINI_AUTO_BARCODE_STATUS 100.vi"("Enum"=enum16{"Read", "Write"}."Write", "error in (no error)"=w1307, "I/P"=w1304) -> ("error out"=w1306:errorcluster)  [unwired: 7 in, 1 out]
              }
            }
            n496 = flat-sequence {
              tunnel: [w1310] -> w1265
              tunnel: w1266 -> [w1310]
              frame #0 {
                # "UPDATE op 100 SCAN sTATUS"
                n497 = global write "DATA LOG.vi" "OP 110 Outputs"(TRUE) -> ()
              }
            }
          }
          frame "DATALOG10" {
            w1324 = T15 2 items=["no dialog", "OK message", "continue or stop message", "OK message + warnings", "continue/stop + warnings"] ("type of dialog (OK msg:1)")
            # "datalog of OP 100"
            n498 = call "PADMINI_AUTO_BARCODE_STRING 100.vi"("Enum"=enum16{"Read", "Write"}."Read", "error in (no error)"=w1312) -> ("error out"=w1318:errorcluster, "Input 2"=w1314:string[])  [unwired: 8 in]
            n499 = call "PADMINI_AUTO_CYCLE VALUE 100.vi"("Enum"=enum16{"Read", "Write"}."Read", "error in (no error)"=w1312) -> ("Input 2"=w1313:sgl[])  [unwired: 8 in, 1 out]
            n500 = Number To Fractional String(number=w1313, precision (6)=i16 2) -> (F-format string=w1315:string[])  [unwired: 2 in]
            n501 = case shown="False" w1329 {
              tunnel: w1330 -> [w1358 w1383]
              tunnel: w1318 -> [w1359 w1382]
              tunnel: [w1361 w1381] -> w1327
              tunnel: [w1360 w1380] -> w1325
              tunnel: w1328 -> [w1357 _]
              tunnel: w1315 -> [w1353 w1365]
              tunnel: w1314 -> [w1350 w1366]
              frame False {
                # "DO TRACEBILITY"
                n502 = Index Array(array=w1350) -> (element #1=w1349:string, element #2=w1335:string, element #3=w1334:string)  [unwired: 3 in]
                n503 = call <vilib>:"Trim Whitespace.vi"("string"=w1349) -> ("trimmed string"=w1351:string)  [unwired: 1 in]
                n504 = Index Array(array=w1353) -> (element #1=w1346:string, element #2=w1345:string, element #3=w1344:string, element #4=w1343:string, element #5=w1342:string, element #6=w1341:string, element #7=w1340:string, element #8=w1339:string, element #9=w1338:string, element #10=w1337:string, element #11=w1336:string)  [unwired: 11 in]
                n505 = local read "SHIFT"() -> (w1348:string)
                n506 = call "PADMINI_SHIFT_DATE.vi"("SHIFT"=w1348) -> ("date/time string"=w1347:string)  [unwired: 10 in]
                n507 = Bundle("date/time string"=w1347, "Input 2"=w1346, "Input 2"=w1345, "Input 2"=w1344, "Input 2"=w1343, "Input 2"=w1342, "Input 2"=w1341, "Input 2"=w1340, "Input 2"=w1339, "Input 2"=w1338, "Input 2"=w1337, "Input 2"=w1336, "Input 2"=w1335, "Input 2"=w1334) -> (w1352:T25)  [unwired: 1 in]
                n508 = Format Into String(format string="Where BARCODE='%s' ", w1351) -> (resulting string=w1355:string)  [unwired: 2 in, 1 out]
                n509 = call <vilib>:"DB Tools Update Data.vi"("condition"=w1355, "data"=w1352, "error in (no error)"=w1359, "columns"=string[] ["OP100_DATE", "OP100_SENSOR_OP_OPEN_V", "OP100_SENSOR_OP_CLOSE_V", "OP100_SENSOR_OP_FULL_CLOSE_V", "OP100_SENSOR_INITIAL_V", "OP100_MOTOR_START_OF_CLOSE_V", "OP100_MOTOR_FULL_CLOSE_V", "OP100_MOTOR_START_BACK_V", "OP100_MOTOR_FULL_OPEN_V", "OP100_RESPONSE_TIME_FWD_msec", "OP100_RESPONSE_TIME_REV_msec", "OP100_MOTOR_PEAK_CURRENT_A", "OP100_FINAL_RESULT", "OP100_CONNECTOR_CAMERA_STATUS"], "table"=w1357, "connection reference"=w1358) -> ("error out"=w1360:errorcluster, "connection reference out"=w1361:T14)  [unwired: 4 in]
              }
              frame True {
                # "TRAC BYPASS"
                n510 = local read "SHIFT"() -> (w1363:string)
                n511 = Index Array(array=w1366) -> (element=w1370:string)  [unwired: 1 in]
                n512 = call "PADMINI_SHIFT_DATE.vi"("SHIFT"=w1363) -> ("date/time string"=w1364:string)  [unwired: 10 in]
                n513 = Index Array(array=w1365) -> (element #1=w1376:string, element #2=w1375:string, element #3=w1362:string, element #4=w1368:string, element #5=w1374:string, element #6=w1369:string, element #7=w1373:string, element #8=w1372:string, element #9=w1371:string)  [unwired: 9 in]
                n514 = Bundle("date/time string"=w1364, "SHIFT"=w1363, "Input 2"=w1376, "Input 2"=w1375, "Input 2"=w1362, "Input 2"=w1362, "Input 2"=w1362, "Input 2"=w1368, "Input 2"=w1374, "Input 2"=w1369, "Input 2"=w1373, "Input 2"=w1372, "Input 2"=w1371, "Input 2"=w1370) -> (w1367:T26)  [unwired: 1 in]
                n515 = To Variant(anything=w1367) -> (Variant=w1379:variant)
                n516 = call <vilib>:"DB Tools Insert Data.vi"("data"=w1379, "error in (no error)"=w1382, "columns"=string[] ["DATE", "SHIFT", "ST10_SENSOR_OP_OPEN_V", "ST10_START_OF_CLOSE_SENSOR_V", "ST10_SENSOR_OP_FULL_CLOSE_V", "ST10_RESPONSE_TIME_FWD", "ST10_RESPONSE_TIME_REV", "ST10_MOTOR_V_START_OF_CLOSE_A", "ST10_MOTOR_V_FULL_CLOSE_B", "ST10_MOTOR_V_START_BACK_C", "ST10_MOTOR_V_FULL_OPEN_D", "ST10_MOTOR_RMS_CURRENT_A", "ST10_FINAL_RST"], "table"="ST10_REPORT", "connection reference"=w1383) -> ("error out"=w1380:errorcluster, "connection reference out"=w1381:T14)  [unwired: 5 in]
              }
            }
            n517 = call <vilib>:"Simple Error Handler.vi"("type of dialog (OK msg:1)"=w1324, "error in (no error)"=w1325) -> ("error out"=w1323:errorcluster)  [unwired: 3 in, 4 out]
            n518 = call <vilib>:"Clear Errors.vi"("error in (no error)"=w1323) -> ("error out"=w1321:errorcluster)  [unwired: 5 in, 1 out]
            n519 = flat-sequence {
              tunnel: [w1333] -> w1311
              tunnel: w1321 -> [w1333]
              frame #0 {
                # "UPDATE op 20 save"
                n520 = global write "DATA LOG.vi" "OP 100 reset"(TRUE) -> ()
              }
            }
          }
          frame "EMERGENCY STOP" {
          }
          frame "STOP" {
            n521 = global read "Global 1.vi" "BARCODE RECIPE"() -> (w1394:string)
            n522 = Bundle("BARCODE RECIPE"=w1394) -> (w1393:cluster{"BARCODE RECIPE":string})  [unwired: 1 in]
            n523 = call <vilib>:"DB Tools Update Data.vi"("data"=w1393, "error in (no error)"=w1399, "columns"=string[] ["PREVIOUS_LOADED_RECIPE"], "table"="BARCODE_RECIPE", "connection reference"=w1397) -> ("error out"=w1398:errorcluster, "connection reference out"=w1396:T14)  [unwired: 5 in]
          }
        }
      }
      frame Error {
        # "Return true in any case that should stop the loop."
      }
    }
    n524 = Unbundle By Name(w130) -> ("OP - 90"=→"OP - 90":T30, "OP - 100"=→"OP - 100":T10, "OP - 110"=→"OP - 110":cluster{"BARCODE":string})
    n525 = Unbundle By Name(w130) -> ("OP - 10"=→"OP - 10":T31, "OP - 20"=→"OP - 20":T5, "OP - 30"=→"OP - 30":T32, "OP - 40"=→"OP - 40":T2)
    n526 = Unbundle By Name(w130) -> ("OP - 50"=→"OP - 50":T1, "OP - 60"=→"OP - 60":T33, "OP - 70"=→"OP - 70":T34, "OP - 80"=→"OP - 80":T35)
    n527 = Wait (ms)(milliseconds to wait=u32 100) -> ()  [unwired: 1 out]
    n528 = call <vilib>:"Simple Error Handler.vi"("error in (no error)"=w124) -> ("error out"=w123:errorcluster)  [unwired: 4 in, 4 out]
  }
  n529 = while {
    shift-right: [w1423] -> w72
    shift-left: w22 -> [w1417]
    shift-right: [w1424] -> w66
    shift-left: w70 -> [w1432]
    stop <- w1422 stop-if-true
    n530 = local read "Shift_change"() -> (w1430:bool)
    n531 = call <vilib>:"Clear Errors.vi"("error in (no error)"=w1417) -> ("error out"=w1408:errorcluster)  [unwired: 5 in, 1 out]
    n532 = call "READ EMERGENCY BIT.vi"("Enum"=enum16{"Read", "Write"}."Read", "error in (no error)"=w1408) -> ("Array Out"=w1420:dbl[])  [unwired: 8 in, 1 out]
    n533 = case shown="True" w1430 {
      tunnel: w1408 -> [w1449 w1462]
      tunnel: [w1450 w1461] -> w1429
      frame False {
        n534 = local read "SHIFT_DATA 2"() -> (w1452:string[])
        n535 = Get Date/Time In Seconds() -> (seconds since 1Jan1904=w1451:timestamp)
        n536 = call "String To Time_4.vi"("error in (no error)"=w1449, "String Array In"=w1452) -> ("error out"=w1448:errorcluster, "Time Stamp Out"=w1447:timestamp[])  [unwired: 8 in]
        "Time Stamp Out 4" <- w1447
        n537 = call "Shift Calculation_4.vi"("error in (no error)"=w1448, "Current Time"=w1451, "Time Stamp Out"=w1447) -> ("error out"=w1446:errorcluster, "Shift"=w1445:i32)  [unwired: 7 in]
        n538 = call <vilib>:"Clear Errors.vi"("error in (no error)"=w1446) -> ()  [unwired: 5 in, 2 out]
        n539 = case shown="4" w1445 {
          tunnel: ["A" "B" "C" "D"] -> w1450
          frame 1, Default {
          }
          frame 2 {
          }
          frame 3 {
          }
          frame 4 {
          }
        }
      }
      frame True {
        n540 = local read "SHIFT_DATA"() -> (w1460:string[])
        n541 = Get Date/Time In Seconds() -> (seconds since 1Jan1904=w1463:timestamp)
        n542 = call "String To Time.vi"("error in (no error)"=w1462, "String Array In"=w1460) -> ("error out"=w1459:errorcluster, "Time Stamp Out"=w1464:timestamp[])  [unwired: 8 in]
        "Time Stamp Out" <- w1464
        n543 = call "Shift Calculation.vi"("error in (no error)"=w1459, "Current Time"=w1463, "Time Stamp Out"=w1464) -> ("error out"=w1458:errorcluster, "Shift"=w1457:i32)  [unwired: 7 in]
        "Shift 4" <- w1457
        n544 = call <vilib>:"Clear Errors.vi"("error in (no error)"=w1458) -> ()  [unwired: 5 in, 2 out]
        n545 = case shown="3" w1457 {
          tunnel: ["A" "B" "C"] -> w1461
          frame 1, Default {
          }
          frame 2 {
          }
          frame 3 {
          }
        }
      }
    }
    "SHIFT" <- w1429
    n546 = Index Array(array=w1420) -> (element=w1419:dbl)  [unwired: 1 in]
    n547 = call "VALUE_CHANGE - ST1_RESULT.vi"("Numeric"=w1419) -> ("Boolean"=w1418:bool)  [unwired: 9 in, 1 out]
    n548 = global write "Global 1.vi" "EMERGENCY STOP"(w1418) -> ()
    n549 = call "Trigger_Loggic.vi"("error in (no error)"=w1408) -> ("error out"=w1413:errorcluster, "Array"=w1433:i32[])  [unwired: 9 in]
    n550 = for {
      tunnel: w1433 -> [w1468] mode=indexing
      shift-right: [w1472] -> w1426
      shift-left: w1432 -> [w1471]
      shift-right: [w1470] -> w1425
      shift-left: w1413 -> [w1469]
      n551 = case shown="0" w1468 {
        tunnel: [w1475 w1480 w1484 w1490 w1495 w1500 w1505 w1510 w1515 w1520 w1525 w1530 w1535 w1540 w1545 w1550 w1555 w1560 w1565 w1570 w1575 w1580 w1585] -> w1472
        tunnel: w1471 -> [w1477 w1482 w1485 w1492 w1497 w1502 w1507 w1512 w1517 w1522 w1527 w1532 w1537 w1542 w1547 w1552 w1557 w1562 w1567 w1572 w1577 w1582 w1587]
        tunnel: [w1474 w1479 w1486 w1489 w1494 w1499 w1504 w1509 w1514 w1519 w1524 w1529 w1534 w1539 w1544 w1549 w1554 w1559 w1564 w1569 w1574 w1579 w1584] -> w1470
        tunnel: w1469 -> [w1476 w1481 w1487 w1491 w1496 w1501 w1506 w1511 w1516 w1521 w1526 w1531 w1536 w1541 w1546 w1551 w1556 w1561 w1566 w1571 w1576 w1581 w1586]
        frame -1, Default {
          # "DEFAULT"
          n552 = Enqueue Element(queue=w1477, element=cluster{"CASE 2":T13} {"CASE 2"=enum."-1"}, error in (no error)=w1476) -> (queue out=w1475:refnum<queue>, error out=w1474:errorcluster)  [unwired: 1 in, 1 out]
        }
        frame 0 {
          # "SCAN BARCODE OP 10"
          n553 = Enqueue Element(queue=w1482, element=cluster{"CASE 2":T13} {"CASE 2"=enum."-1"}, error in (no error)=w1481) -> (queue out=w1480:refnum<queue>, error out=w1479:errorcluster)  [unwired: 1 in, 1 out]
        }
        frame 1 {
          # "DATALOG OF OP 10"
          n554 = Enqueue Element(queue=w1485, element=cluster{"CASE 2":T13} {"CASE 2"=enum."SCAN1"}, error in (no error)=w1487) -> (queue out=w1484:refnum<queue>, error out=w1486:errorcluster)  [unwired: 1 in, 1 out]
        }
        frame 2 {
          # "SCAN BARCODE OP 20"
          n555 = Enqueue Element(queue=w1492, element=cluster{"CASE 2":T13} {"CASE 2"=enum."SCAN2"}, error in (no error)=w1491) -> (queue out=w1490:refnum<queue>, error out=w1489:errorcluster)  [unwired: 1 in, 1 out]
        }
        frame 3 {
          # "DATALOG OF OP 20"
          n556 = Enqueue Element(queue=w1497, element=cluster{"CASE 2":T13} {"CASE 2"=enum."DATALOG2"}, error in (no error)=w1496) -> (queue out=w1495:refnum<queue>, error out=w1494:errorcluster)  [unwired: 1 in, 1 out]
        }
        frame 4 {
          # "SCAN BARCODE OP 30"
          n557 = Enqueue Element(queue=w1502, element=cluster{"CASE 2":T13} {"CASE 2"=enum."SCAN3"}, error in (no error)=w1501) -> (queue out=w1500:refnum<queue>, error out=w1499:errorcluster)  [unwired: 1 in, 1 out]
        }
        frame 5 {
          # "DATALOG OF OP 30"
          n558 = Enqueue Element(queue=w1507, element=cluster{"CASE 2":T13} {"CASE 2"=enum."DATALOG3"}, error in (no error)=w1506) -> (queue out=w1505:refnum<queue>, error out=w1504:errorcluster)  [unwired: 1 in, 1 out]
        }
        frame 6 {
          # "SCAN BARCODE OP 40"
          n559 = Enqueue Element(queue=w1512, element=cluster{"CASE 2":T13} {"CASE 2"=enum."SCAN4"}, error in (no error)=w1511) -> (queue out=w1510:refnum<queue>, error out=w1509:errorcluster)  [unwired: 1 in, 1 out]
        }
        frame 7 {
          # "DATALOG OF OP 40"
          n560 = Enqueue Element(queue=w1517, element=cluster{"CASE 2":T13} {"CASE 2"=enum."DATALOG4"}, error in (no error)=w1516) -> (queue out=w1515:refnum<queue>, error out=w1514:errorcluster)  [unwired: 1 in, 1 out]
        }
        frame 8 {
          # "SCAN BARCODE OP 50"
          n561 = Enqueue Element(queue=w1522, element=cluster{"CASE":T13} {"CASE"=enum."SCAN5"}, error in (no error)=w1521) -> (queue out=w1520:refnum<queue>, error out=w1519:errorcluster)  [unwired: 1 in, 1 out]
        }
        frame 9 {
          # "DATALOG OF OP 50"
          n562 = Enqueue Element(queue=w1527, element=cluster{"CASE":T13} {"CASE"=enum."DATALOG5"}, error in (no error)=w1526) -> (queue out=w1525:refnum<queue>, error out=w1524:errorcluster)  [unwired: 1 in, 1 out]
        }
        frame 10 {
          # "SCAN BARCODE OP 60"
          n563 = Enqueue Element(queue=w1532, element=cluster{"CASE 2":T13} {"CASE 2"=enum."SCAN6"}, error in (no error)=w1531) -> (queue out=w1530:refnum<queue>, error out=w1529:errorcluster)  [unwired: 1 in, 1 out]
        }
        frame 11 {
          # "DATALOG OF OP 60"
          n564 = Enqueue Element(queue=w1537, element=cluster{"CASE 2":T13} {"CASE 2"=enum."DATALOG6"}, error in (no error)=w1536) -> (queue out=w1535:refnum<queue>, error out=w1534:errorcluster)  [unwired: 1 in, 1 out]
        }
        frame 12 {
          # "SCAN BARCODE OP 70"
          n565 = Enqueue Element(queue=w1542, element=cluster{"CASE 2":T13} {"CASE 2"=enum."SCAN7"}, error in (no error)=w1541) -> (queue out=w1540:refnum<queue>, error out=w1539:errorcluster)  [unwired: 1 in, 1 out]
        }
        frame 13 {
          # "DATALOG OF OP 70"
          n566 = Enqueue Element(queue=w1547, element=cluster{"CASE 2":T13} {"CASE 2"=enum."DATALOG7"}, error in (no error)=w1546) -> (queue out=w1545:refnum<queue>, error out=w1544:errorcluster)  [unwired: 1 in, 1 out]
        }
        frame 14 {
          # "SCAN BARCODE 80"
          n567 = Enqueue Element(queue=w1552, element=cluster{"CASE 2":T13} {"CASE 2"=enum."SCAN8"}, error in (no error)=w1551) -> (queue out=w1550:refnum<queue>, error out=w1549:errorcluster)  [unwired: 1 in, 1 out]
        }
        frame 15 {
          # "DATALOG OF OP 80"
          n568 = Enqueue Element(queue=w1557, element=cluster{"CASE 2":T13} {"CASE 2"=enum."DATALOG8"}, error in (no error)=w1556) -> (queue out=w1555:refnum<queue>, error out=w1554:errorcluster)  [unwired: 1 in, 1 out]
        }
        frame 16 {
          # "SCAN BARCODE OP 90"
          n569 = Enqueue Element(queue=w1562, element=cluster{"CASE 2":T13} {"CASE 2"=enum."SCAN9"}, error in (no error)=w1561) -> (queue out=w1560:refnum<queue>, error out=w1559:errorcluster)  [unwired: 1 in, 1 out]
        }
        frame 17 {
          # "DATALOG OF OP 90"
          n570 = Enqueue Element(queue=w1567, element=cluster{"CASE 2":T13} {"CASE 2"=enum."DATALOG9"}, error in (no error)=w1566) -> (queue out=w1565:refnum<queue>, error out=w1564:errorcluster)  [unwired: 1 in, 1 out]
        }
        frame 18 {
          # "SCAN BARCODE OP 100"
          n571 = Enqueue Element(queue=w1572, element=cluster{"CASE 2":T13} {"CASE 2"=enum."SCAN10"}, error in (no error)=w1571) -> (queue out=w1570:refnum<queue>, error out=w1569:errorcluster)  [unwired: 1 in, 1 out]
        }
        frame 19 {
          # "DATALOG OF OP 100"
          n572 = Enqueue Element(queue=w1577, element=cluster{"CASE 2":T13} {"CASE 2"=enum."DATALOG10"}, error in (no error)=w1576) -> (queue out=w1575:refnum<queue>, error out=w1574:errorcluster)  [unwired: 1 in, 1 out]
        }
        frame 20 {
          # "SCAN BARCODE OP 110"
          n573 = Enqueue Element(queue=w1582, element=cluster{"CASE 2":T13} {"CASE 2"=enum."SCAN11"}, error in (no error)=w1581) -> (queue out=w1580:refnum<queue>, error out=w1579:errorcluster)  [unwired: 1 in, 1 out]
        }
        frame 21 {
          # "DATALOG OF OP 110"
          n574 = Enqueue Element(queue=w1587, element=cluster{"CASE 2":T13} {"CASE 2"=enum."DATALOG11"}, error in (no error)=w1586) -> (queue out=w1585:refnum<queue>, error out=w1584:errorcluster)  [unwired: 1 in, 1 out]
        }
      }
    }
    n575 = Wait (ms)(milliseconds to wait=u32 50) -> ()  [unwired: 1 out]
    n576 = global read "Global 1.vi" "PLC COMM"() -> (→"PLC COM.":bool)
    n577 = global read "Global 1.vi" "PLC 1"() -> (→"OP 10 & 20":bool)
    n578 = global read "Global 1.vi" "PLC 2"() -> (→"OP 30":bool)
    n579 = global read "Global 1.vi" "PLC 3"() -> (→"OP 40":bool)
    n580 = case shown="False" "stop 2" {
      tunnel: w1426 -> [w1436 w1442]
      tunnel: [w1436 w1441] -> w1424
      tunnel: w1425 -> [w1435 w1440]
      tunnel: [w1435 w1439] -> w1423
      tunnel: [FALSE TRUE] -> w1422
      frame False {
      }
      frame True {
        n581 = Flush Queue(queue=w1442, error in (no error)=w1440) -> (queue out=w1444:refnum<queue>, error out=w1443:errorcluster)  [unwired: 1 out]
        n582 = Enqueue Element(queue=w1444, element=cluster{"CASE 2":T13} {"CASE 2"=enum."STOP"}, error in (no error)=w1443) -> (queue out=w1441:refnum<queue>, error out=w1439:errorcluster)  [unwired: 1 in, 1 out]
      }
    }
    "stop" <- w1422
    n583 = global read "Global 1.vi" "PLC 4"() -> (→"OP 50":bool)
    n584 = global read "Global 1.vi" "PLC 5"() -> (→"OP 60":bool)
    n585 = global read "Global 1.vi" "PLC 7"() -> (→"OP 90 -100 - 110":bool)
    n586 = global read "Global 1.vi" "PLC 6"() -> (→"OP 70 & 80":bool)
  }
  n587 = Release Queue(queue=w66, error in (no error)=w72) -> (error out=w49:errorcluster)  [unwired: 1 in, 2 out]
  n588 = call <vilib>:"Clear Errors.vi"("error in (no error)"=w68) -> ("error out"=w53:errorcluster)  [unwired: 5 in, 1 out]
  n589 = call <vilib>:"DB Tools Close Connection.vi"("error in (no error)"=w53, "connection reference"=w67) -> ("error out"=w50:errorcluster)  [unwired: 5 in]
  n590 = Merge Errors(w49, w50) -> (w51:errorcluster)
  n591 = call <vilib>:"Simple Error Handler.vi"("error in (no error)"=w51) -> ("error out"=w46:errorcluster)  [unwired: 4 in, 4 out]
  n592 = call <vilib>:"Clear Errors.vi"("error in (no error)"=w46) -> ("error out"=w52:errorcluster)  [unwired: 5 in, 1 out]
  n593 = flat-sequence {
    tunnel: w52 -> [w1590]
    tunnel: [w1590] -> w54
    frame #0 {
      n594 = global write "Global 1.vi" "REMOVE VI"(TRUE ("remove_VI")) -> ()
      n595 = global write "DATA LOG.vi" "Auto Cycle On"(FALSE) -> ()
    }
  }
  n596 = property class="App"(error in=w54) -> (error out=w56:errorcluster, "App.Kind"=w55:T36)  [unwired: 1 in, 1 out]
  n597 = case shown="\"Run Time System\"" w55 {
    tunnel: [w1591 w1593] -> w57
    tunnel: w56 -> [w1591 w1592]
    frame "Development System", Default {
    }
    frame "Run Time System" {
      n598 = invoke class="VI" method="FP.Close"(error in=w1592) -> (error out=w1593:errorcluster)  [unwired: 2 in, 2 out]
    }
  }
  "error out 2" <- w57
